vi "PSUSettingsMenu.vi"(8 "error in (no error)":errorcluster, 9 "PSU Calc":T1={"Low speed (km/s)"=2000.0, "High speed (km/s)"=3000.0, "Window (Delta-T)"=0.0, "Lower Cutoff"=0.0, "Multiplier"=0, "Low Charge (fC)"=2000.0, "High Charge (fC)"=2000.0, "High Mass (kg)"=2000.0, "Low Mass (kg)"=2000.0, "High Radius (µm) "=0.0, "Low Radius (µm)"=2000.0, "Exp. Voltage (MV)"=2000.0} {"Exp. Voltage (MV)" step=0.01 format="%#.6f"; "Window (Delta-T)" step=1.0 format="%#.0f"; "High Radius (µm)" min=0.0 max=1000.0; "High Mass (kg)" min=0.0 max=1.0; "High Charge (fC)" min=0.0 max=1000000000000.0; "High speed (km/s)" min=0.0 max=299790.0; "Low speed (km/s)" min=0.0 max=299790.0; "Low Charge (fC)" min=0.0 max=1000000000000.0; "Low Mass (kg)" min=0.0 max=1.0; "Low Radius (µm)" min=0.0 max=299792000.0; "Lower Cutoff" step=1.0 format="%#.0f"; "Multiplier" items=["1k", "10k"]}, 10 "sub vi?":bool, 11 "Enable":bool=TRUE) -> (0 "error out":errorcluster, 1 "OK":bool, 3 "Cancel 2":bool caption="Cancel")   [LabVIEW 2013]
doc: "Displays a standard dialog box that prompts users to enter information, such as a user name and password.\n--------------------\n\nThis Express VI is configured as follows:\n\nMessage to Display to the User:Please Enter Experiment Settings Information For Database Storage.\nThe inputs are: \nNumber: Please Enter Group ID\nText Entry Box: Please Enter Tags:\nText Entry Box: Please Enter Experiment Description:"
uses:
  Controls/PSU Calc.ctl
  <vilib>/Utility/miscctls.llb/LVPointTypeDef.ctl
  Global Variables/PSU updated.vi
  Sub-Polymorphic/post_psu.vi
  <vilib>/addons/database/_DB Variant To Data/Database Variant To Data.xnode
panel:
  in  "Accept All Particles":bool caption="OK2"
  out "Dust Density\n(g/cc)":dbl
  in  "Variable 2":enum32{"Velocity", "Charge", "Mass"}(radio)
  in  "Variable 1":enum32{"Velocity", "Charge", "Mass"}(radio)
  in  "PSU update":bool caption="OK2"
  in  "Cancel":bool
  in  "OK1":bool
  # "Please Enter PSU Settings For Storage in the CCLDAS Database."
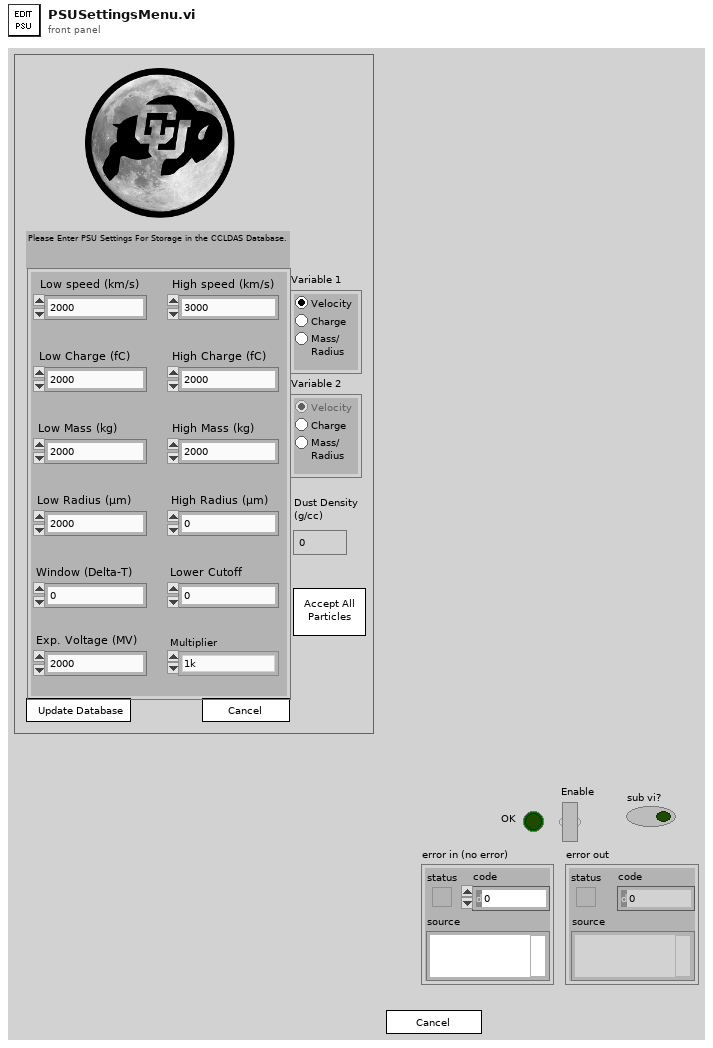
[diagram p1: front panel]
types:
  T1 = typedef "PSU Calc.ctl" = cluster{"Low speed (km/s)":dbl, "High speed (km/s)":dbl, "Window (Delta-T)":dbl, "Lower Cutoff":dbl, "Multiplier":u16, "Low Charge (fC)":dbl, "High Charge (fC)":dbl, "High Mass (kg)":dbl, "Low Mass (kg)":dbl, "High Radius (µm) ":dbl, "Low Radius (µm)":dbl, "Exp. Voltage (MV)":dbl}
  T2 = typedef "LVPointTypeDef.ctl" = cluster{"Horizontal":i16, "Vertical":i16}
  T3 = enum32{"Invalid", "Standard", "Closed", "Hidden", "Minimized", "Maximized"}
  T4 = enum8{"Enabled", "Disabled", "Disabled and Grayed Out"}
  T5 = cluster{"Integer Timestamp":i64, "Max Velocity":dbl, "Min Velocity":dbl, "Max Charge":dbl, "Min Charge":dbl, "Max Mass":dbl, "Min Mass":dbl, "Variable 1":enum8{"Velocity", "Charge", "Mass"}, "Variable 2":enum8{"Velocity", "Charge", "Mass"}}
  T6 = cluster{"Integer Timestamp":dbl, "Max Velocity":dbl, "Min Velocity":dbl, "Max Charge":dbl, "Min Charge":dbl, "Max Mass":dbl, "Min Mass":dbl, "Variable 1":enum32{"Velocity", "Charge", "Mass", "Radius"}, "Variable 2":enum32{"Velocity", "Charge", "Mass", "Radius"}}
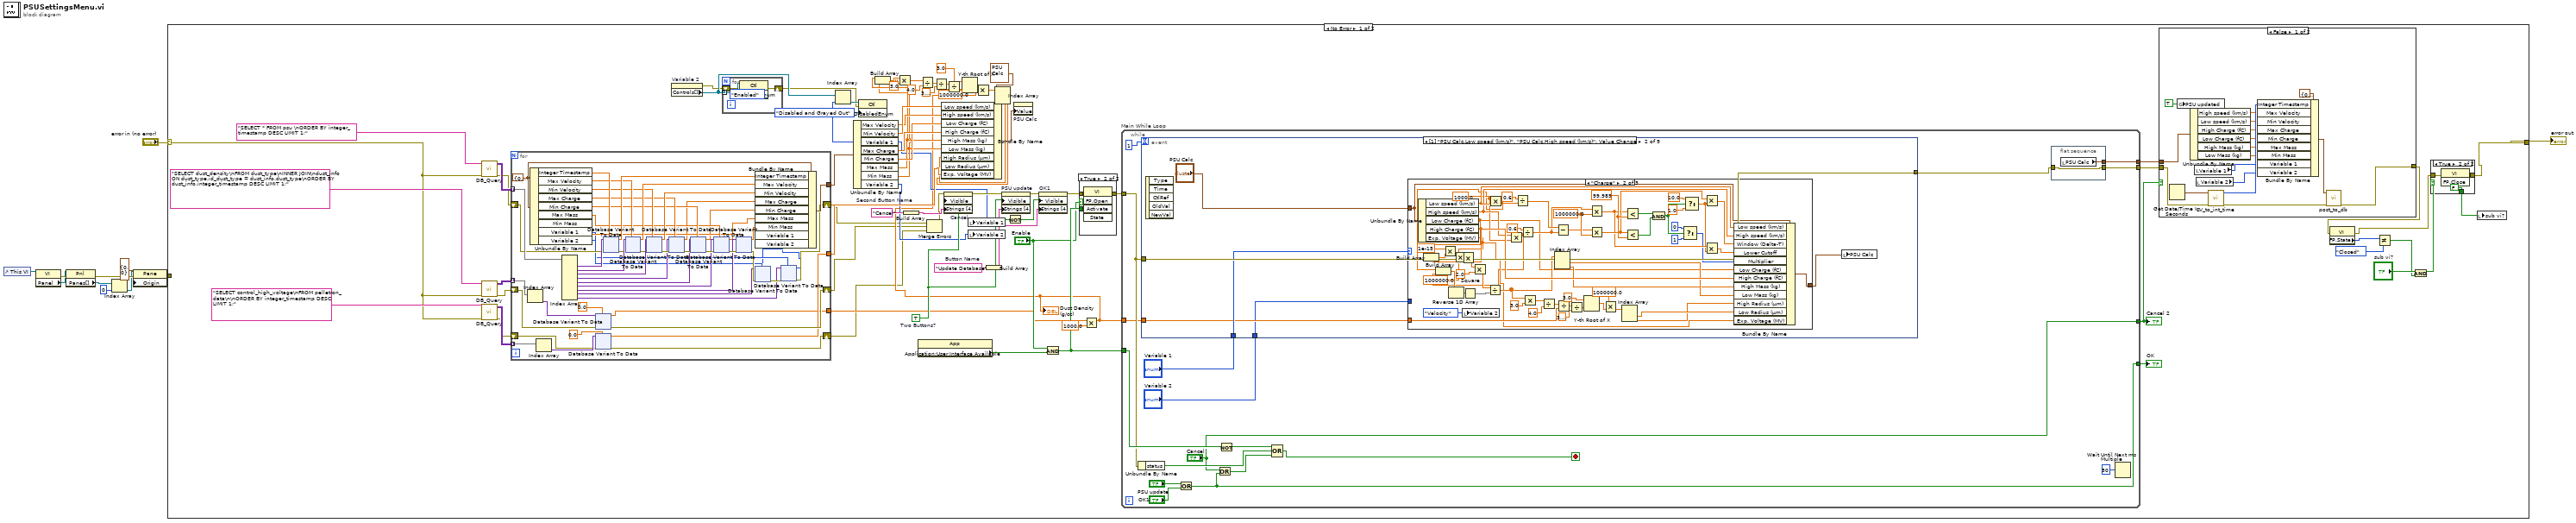
[diagram p0: block diagram]
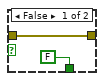
[diagram p2: hidden frame]
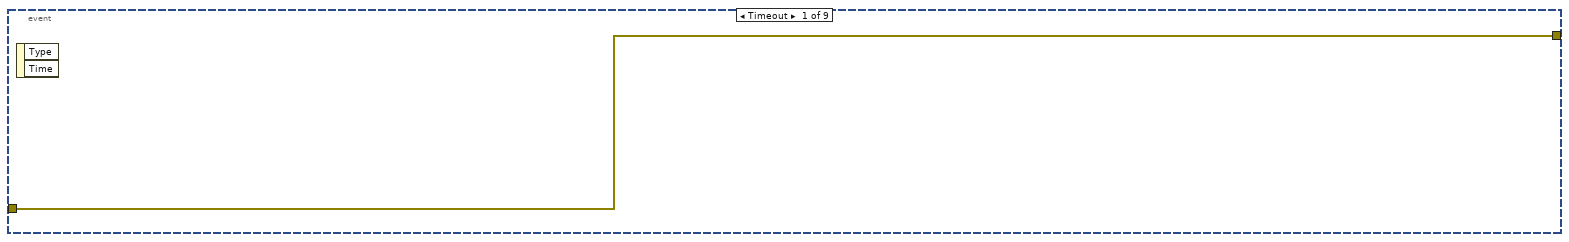
[diagram p5: hidden frame]
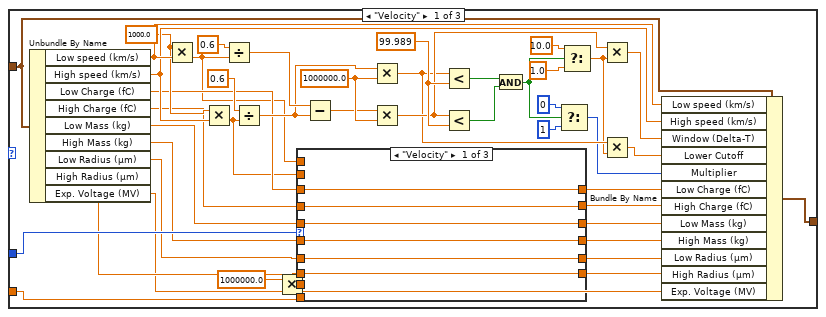
[diagram p6: hidden frame]
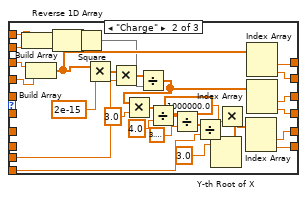
[diagram p7: hidden frame]
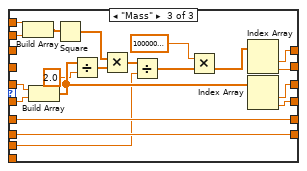
[diagram p8: hidden frame]
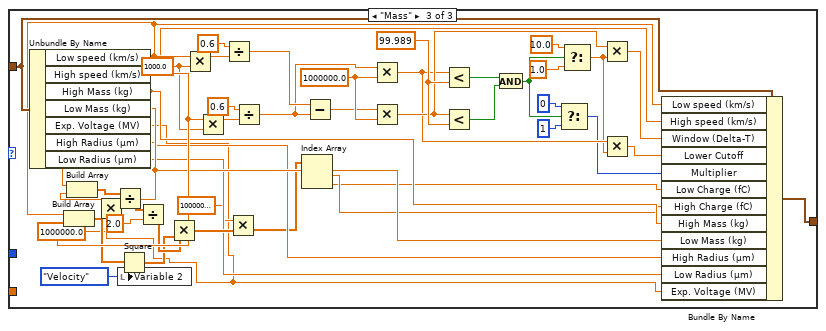
[diagram p9: hidden frame]
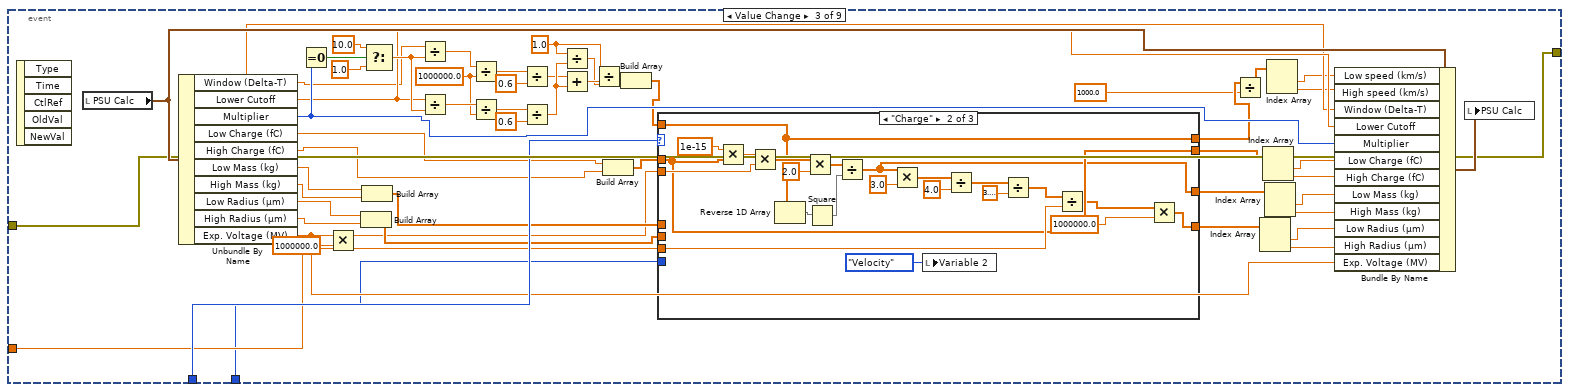
[diagram p10: hidden frame]
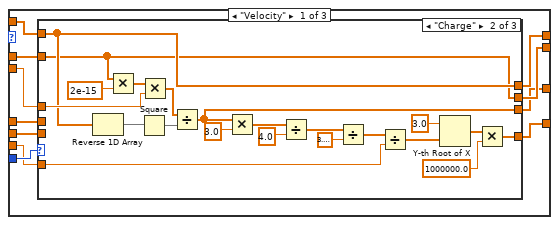
[diagram p11: hidden frame]
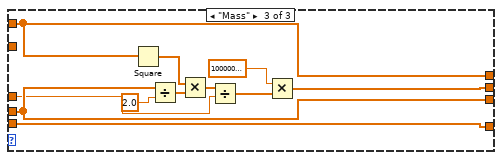
[diagram p13: hidden frame]
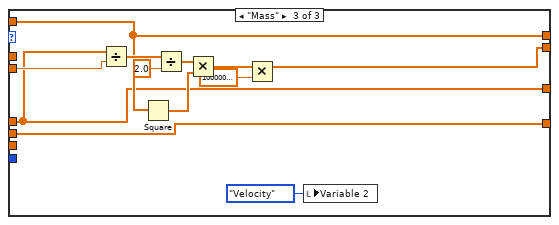
[diagram p14: hidden frame]
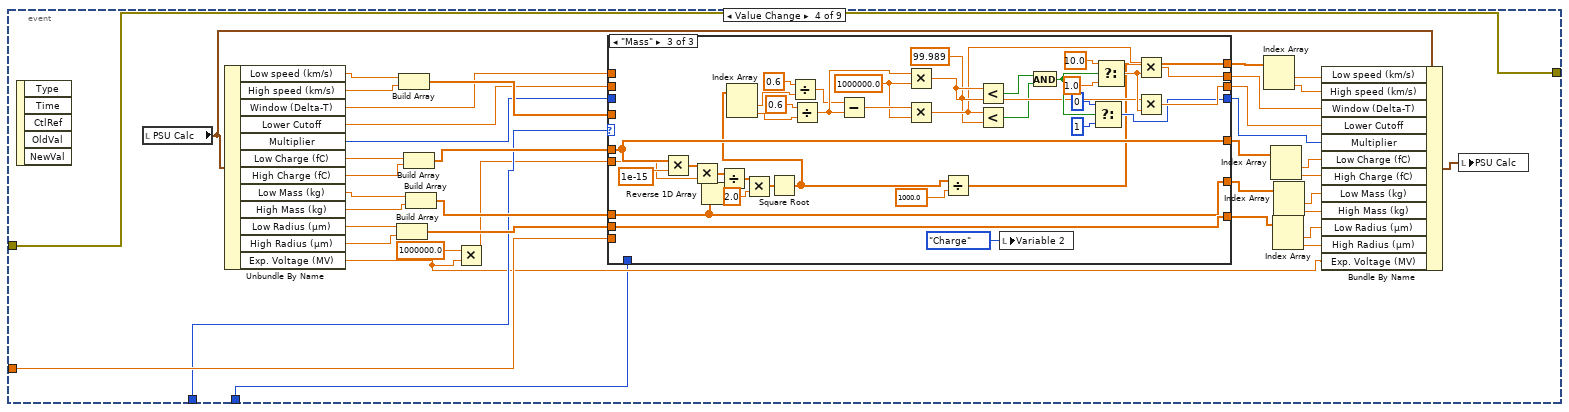
[diagram p15: hidden frame]
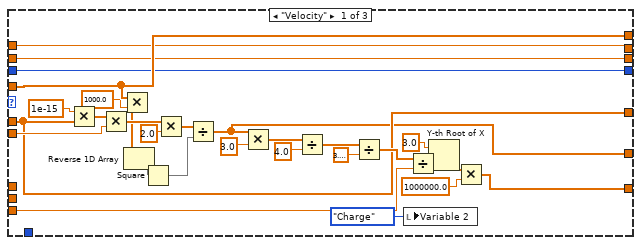
[diagram p16: hidden frame]
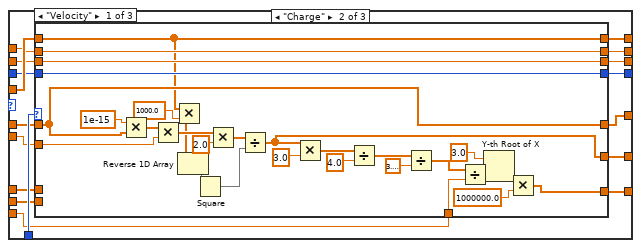
[diagram p17: hidden frame]
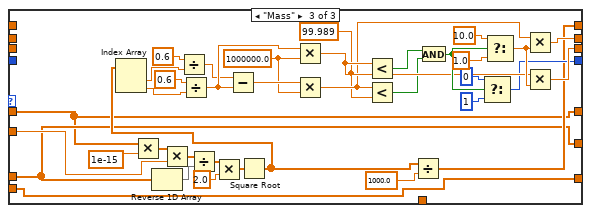
[diagram p19: hidden frame]
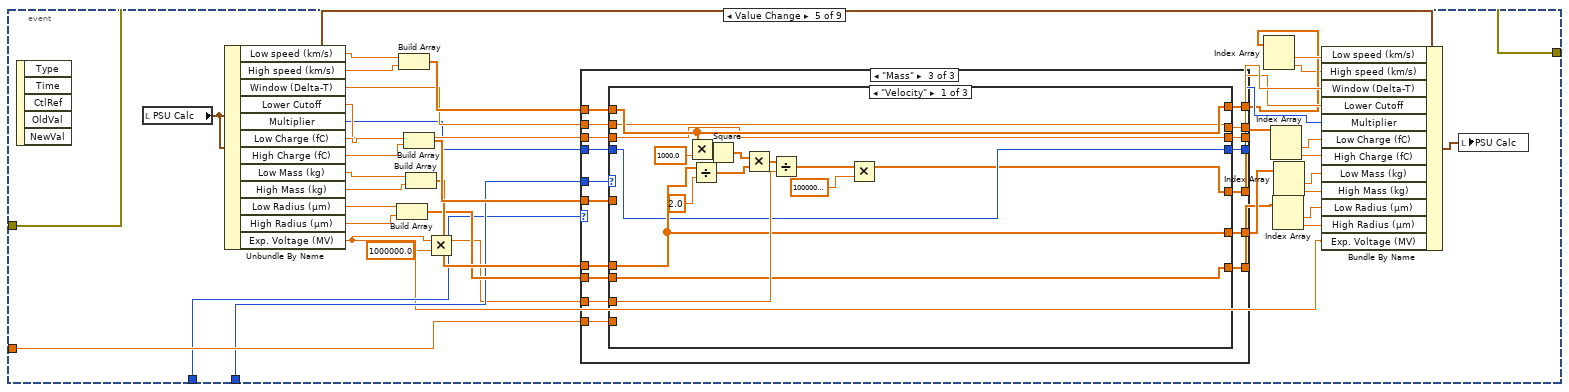
[diagram p20: hidden frame]
diagram:
  n1 = control-ref of="This VI"() -> (w9:refnum<vi>)
  n2 = property class="VI"(reference=w9) -> (error out=w8:errorcluster, "Panel"=w7:refnum<vi>)  [unwired: 1 in, 1 out]
  n3 = property class="Pnl"(reference=w7, error in=w8) -> (error out=w6:errorcluster, "Panes[]"=w5:refnum<vi>[])  [unwired: 1 out]
  n4 = Index Array(array=w5, index=0) -> (element=w3:refnum<vi>)
  n5 = property class="Pane"(reference=w3, error in=w6, "Origin"=T2 {"Horizontal"=0, "Vertical"=0}) -> (error out=w1:errorcluster)  [unwired: 1 out]
  n6 = case shown="No Error" "error in (no error)" {
    selector: "error in (no error)" -> [w13 w1720]
    tunnel: [w36 w1720] -> w10
    tunnel: w1 -> [_ _]
    frame No Error {
      w80 = "Cancel"  # Second Button Name
      w82 = "Update Database"  # Button Name
      w74 = TRUE  # Two Buttons?
      n7 = call "DB_Query.vi"("error in (no error)"=w13, "Parameterized Query"="SELECT * FROM psu \nORDER BY integer_timestamp DESC LIMIT 1;" ("SQL query")) -> ("error out"=w17:errorcluster, "Results"=w19:variant[][])  [unwired: 7 in, 1 out]
      n8 = call "DB_Query.vi"("error in (no error)"=w13, "Parameterized Query"="SELECT dust_density\nFROM dust_type\nINNER JOIN\ndust_info ON dust_type.id_dust_type = dust_info.dust_type\nORDER BY dust_info.integer_timestamp DESC LIMIT 1;" ("SQL query")) -> ("error out"=w18:errorcluster, "Results"=w21:variant[][])  [unwired: 7 in, 1 out]
      n9 = call "DB_Query.vi"("error in (no error)"=w13, "Parameterized Query"="SELECT control_high_voltage\nFROM pelletron_data\n\nORDER BY integer_timestamp DESC LIMIT 1;" ("SQL query")) -> ("error out"=w12:errorcluster, "Results"=w23:variant[][])  [unwired: 7 in, 1 out]
      n10 = for {
        tunnel: w19 -> [w168] mode=indexing
        shift-right: [w127] -> w14
        shift-left: w17 -> [w164]
        tunnel: [w163] -> w73
        tunnel: w21 -> [w137] mode=indexing
        shift-right: [w131] -> w15
        shift-left: w18 -> [w132]
        tunnel: w23 -> [w136] mode=indexing
        shift-right: [w130] -> w16
        shift-left: w12 -> [w133]
        tunnel: [w119] -> w60
        tunnel: [w117] -> w26
        w158 = T6 {"Integer Timestamp"=0.0, "Max Velocity"=0.0, "Min Velocity"=0.0, "Max Charge"=0.0, "Min Charge"=0.0, "Max Mass"=0.0, "Min Mass"=0.0, "Variable 1"=enum."Velocity", "Variable 2"=enum."Velocity"} ("PSU settings")
        n11 = Index Array(array=w137) -> (element=w135:variant)  [unwired: 1 in]
        n12 = Unbundle By Name(w158) -> ("Integer Timestamp"=w162:dbl, "Max Velocity"=w159:dbl, "Min Velocity"=w156:dbl, "Max Charge"=w145:dbl, "Min Charge"=w144:dbl, "Max Mass"=w143:dbl, "Min Mass"=w142:dbl, "Variable 1"=w124:enum32{"Velocity", "Charge", "Mass", "Radius"}, "Variable 2"=w123:enum32{"Velocity", "Charge", "Mass", "Radius"})
        n13 = Index Array(array=w136) -> (element=w134:variant)  [unwired: 1 in]
        n14 = Index Array(array=w168) -> (element #1=w167:variant, element #2=w166:variant, element #3=w157:variant, element #4=w150:variant, element #5=w149:variant, element #6=w148:variant, element #7=w146:variant, element #8=w126:variant, element #9=w125:variant)  [unwired: 9 in]
        n15 = xnode "Database Variant To Data"("database variant"=w135, "error in (no error)"=w132, "type"=0.0) -> ("data"=w117:dbl, "error out"=w131:errorcluster)
        n16 = xnode "Database Variant To Data"("database variant"=w134, "error in (no error)"=w133, "type"=0.0) -> ("data"=w119:dbl, "error out"=w130:errorcluster)
        n17 = xnode "Database Variant To Data"("database variant"=w167, "error in"=w164, "type"=w162) -> ("data"=w161:dbl, "error out"=w165:errorcluster)
        n18 = xnode "Database Variant To Data"("database variant"=w166, "error in"=w165, "type"=w159) -> ("data"=w160:dbl, "error out"=w154:errorcluster)
        n19 = xnode "Database Variant To Data"("database variant"=w157, "error in"=w154, "type"=w156) -> ("data"=w155:dbl, "error out"=w151:errorcluster)
        n20 = xnode "Database Variant To Data"("database variant"=w150, "error in (no error)"=w151, "type"=w145) -> ("data"=w141:dbl, "error out"=w153:errorcluster)
        n21 = xnode "Database Variant To Data"("database variant"=w149, "error in (no error)"=w153, "type"=w144) -> ("data"=w140:dbl, "error out"=w152:errorcluster)
        n22 = xnode "Database Variant To Data"("database variant"=w148, "error in (no error)"=w152, "type"=w143) -> ("data"=w139:dbl, "error out"=w147:errorcluster)
        n23 = xnode "Database Variant To Data"("database variant"=w146, "error in (no error)"=w147, "type"=w142) -> ("data"=w138:dbl, "error out"=w128:errorcluster)
        n24 = xnode "Database Variant To Data"("database variant"=w126, "error in (no error)"=w128, "type"=w124) -> ("data"=w122:enum32{"Velocity", "Charge", "Mass", "Radius"}, "error out"=w129:errorcluster)
        n25 = xnode "Database Variant To Data"("database variant"=w125, "error in (no error)"=w129, "type"=w123) -> ("data"=w121:enum32{"Velocity", "Charge", "Mass", "Radius"}, "error out"=w127:errorcluster)
        n26 = Bundle By Name(cluster=w158, "Integer Timestamp"=w161, "Max Velocity"=w160, "Min Velocity"=w155, "Max Charge"=w141, "Min Charge"=w140, "Max Mass"=w139, "Min Mass"=w138, "Variable 1"=w122, "Variable 2"=w121) -> (w163:T6)
      }
      n27 = property on="Variable 2" class="RadioBtnsControl (strict)"() -> (error out=w42:errorcluster, "Controls[]"=w43:refnum<vi>[])  [unwired: 2 in, 1 out]
      n28 = for {
        tunnel: w43 -> [w98] mode=indexing
        shift-right: [w95] -> w41
        shift-left: w42 -> [w97]
        n29 = property class="Ctl"(reference=w98, error in=w97, "DisabledEnum"=T4."Enabled" ("Disabled")) -> (error out=w95:errorcluster)  [unwired: 1 out]
      }
      n30 = Unbundle By Name(w73) -> ("Max Velocity"=w69:dbl, "Min Velocity"=w70:dbl, "Variable 1"=w40:enum32{"Velocity", "Charge", "Mass", "Radius"}, "Max Charge"=w62:dbl, "Min Charge"=w61:dbl, "Max Mass"=w59:dbl, "Min Mass"=w58:dbl, "Variable 2"=w39:enum32{"Velocity", "Charge", "Mass", "Radius"})
      n31 = Index Array(array=w43, index=w40) -> (element=w64:refnum<vi>)
      n32 = property class="Ctl"(reference=w64, error in=w41, "DisabledEnum"=T4."Disabled and Grayed Out" ("Disabled")) -> ()  [unwired: 2 out]
      n33 = Build Array(w59, w58) -> (w57:dbl[])
      n34 = Multiply(x=w57, y=3.0 ("Min Mass")) -> (x*y=w55:dbl[])
      n35 = Build Array(w80) -> (w79:string[])
      n36 = property class="App"() -> ("Application:User Interface Available"=w84:bool)  [unwired: 2 in, 2 out]
      n37 = Divide(x=w55, y=4.0 ("Min Mass")) -> (x/y=w53:dbl[])
      n38 = Merge Errors(w14, w15, w16) -> (w65:errorcluster)
      n39 = Divide(x=w53, y=3.141592653589793) -> (x/y=w51:dbl[])
      n40 = property on="Cancel" class="Bool"(error in=w65, "Visible"=w74, "Strings [4]"=w79) -> (error out=w77:errorcluster)  [unwired: 1 in, 1 out]
      n41 = local write "Variable 1"(w40) -> ()
      n42 = local write "Variable 2"(w39) -> ()
      n43 = Build Array(w82) -> (w81:string[])
      n44 = property on="PSU update" class="Bool"(error in=w77, "Visible"=w74, "Strings [4]"=w81) -> (error out=w78:errorcluster)  [unwired: 1 in, 1 out]
      n45 = Not(x=w74) -> (.not. x?=w76:bool)
      n46 = property on="OK1" class="Bool"(error in=w78, "Visible"=w76, "Strings [4]"=w81) -> (error out=w83:errorcluster)  [unwired: 1 in, 1 out]
      n47 = And(x="Enable", y=w84) -> (x .and. y?=w38:bool)
      n48 = case shown="True" "Enable" {
        tunnel: [w91 w94] -> w85
        tunnel: w83 -> [w91 w93]
        tunnel: w38 -> [_ w92]
        frame False {
        }
        frame True {
          n49 = invoke class="VI" method="FP.Open"(error in=w93, "Activate"=w92) -> (error out=w94:errorcluster)  [unwired: 3 in, 4 out]
        }
      }
      n50 = Multiply(x=w26, y=1000.0) -> (x*y=w25:dbl)
      "Dust Density\n(g/cc)" <- w25
      n51 = Divide(x=w51, y=w25) -> (x/y=w50:dbl[])
      n52 = Y-th Root of X(1:w50, 2:3.0 ("Min Mass")) -> (0:w46:dbl[])
      n53 = Multiply(x=w46, y=1000000.0 ("Min Mass")) -> (x*y=w45:dbl[])
      n54 = Index Array(array=w45) -> (element #1=w49:dbl, element #2=w48:dbl)  [unwired: 2 in]
      n55 = Bundle By Name(cluster=T1 {"Low speed (km/s)"=2000.0, "High speed (km/s)"=3000.0, "Window (Delta-T)"=0.0, "Lower Cutoff"=0.0, "Multiplier"=0, "Low Charge (fC)"=0.0, "High Charge (fC)"=0.0, "High Mass (kg)"=0.0, "Low Mass (kg)"=0.0, "High Radius (µm) "=0.0, "Low Radius (µm)"=0.0, "Exp. Voltage (MV)"=0.0} ("PSU Calc"), "Low speed (km/s)"=w70, "High speed (km/s)"=w69, "Low Charge (fC)"=w61, "High Charge (fC)"=w62, "High Mass (kg)"=w59, "Low Mass (kg)"=w58, "High Radius (µm)"=w49, "Low Radius (µm)"=w48, "Exp. Voltage (MV)"=w60) -> (w72:T1)
      n56 = property on="PSU Calc" class="Clust (strict)"("Value"=w72) -> ()  [unwired: 2 in, 2 out]
      n57 = while "Main While Loop" {
        tunnel: [w536] -> w75
        tunnel: w38 -> [w534]
        tunnel: w85 -> [w528]
        tunnel: [w526] -> w67
        tunnel: ["Cancel"] -> w68
        tunnel: [w524] -> w66
        tunnel: w25 -> [w522]
        stop <- w530 stop-if-true
        n58 = Unbundle By Name(w528) -> ("status"=w531:bool)
        n59 = event shown="[1] \"PSU Calc.Low speed (km/s)\", \"PSU Calc.High speed (km/s)\": Value Change" {
          selector: _ -> [_ _ _ _ _ _ _ _ _]
          dyn-events: _ -> [_ _ _ _ _ _ _ _ _]
          timeout: 1 -> [_ _ _ _ _ _ _ _ _]
          tunnel: w528 -> [w541 w546 w804 w892 w1084 w1356 w1367 w1535 w1719]
          tunnel: [w541 w546 w804 w892 w1084 w1348 w1367 w1535 w1697] -> w525
          tunnel: "Variable 1" -> [_ w544 w785 w893 w1085 _ w1381 w1551 _]
          tunnel: w522 -> [_ w543 w778 w912 w1105 _ w1373 w1544 _]
          tunnel: "Variable 2" -> [_ w542 w754 w888 w1086 w1352 w1363 w1531 _]
          event Timeout {
            n60 = event-data() -> ()  [unwired: 1 in, 2 out]
          }
          event Value Change {
            n61 = event-data() -> ()  [unwired: 1 in, 5 out]
            n62 = case shown="\"Charge\"" w544 {
              tunnel: [w591 w707 w753] -> w547
              tunnel: "PSU Calc" -> [w590 w706 w752]
              tunnel: w543 -> [w550 w668 _]
              tunnel: w542 -> [w566 _ _]
              frame "Velocity" {
                w567 = 1000.0 ("x")
                w581 = 99.989
                w583 = 1000000.0 ("y")
                n63 = Unbundle By Name(w590) -> ("Low speed (km/s)"=w572:dbl, "High speed (km/s)"=w568:dbl, "Low Charge (fC)"=w565:dbl, "High Charge (fC)"=w563:dbl, "Low Mass (kg)"=w561:dbl, "High Mass (kg)"=w560:dbl, "Low Radius (µm)"=w557:dbl, "High Radius (µm)"=w555:dbl, "Exp. Voltage (MV)"=w553:dbl)
                n64 = Multiply(x=w567, y=w572) -> (x*y=w551:dbl)
                n65 = Multiply(x=w567, y=w568) -> (x*y=w552:dbl)
                n66 = Divide(x=0.6, y=w551) -> (x/y=w585:dbl)
                n67 = Divide(x=0.6, y=w552) -> (x/y=w584:dbl)
                n68 = Multiply(x=1000000.0, y=w553) -> (x*y=w549:dbl)
                n69 = case shown="\"Velocity\"" w566 {
                  tunnel: w565 -> [w597 w625 _]
                  tunnel: [w597 w624 w642] -> w564
                  tunnel: w563 -> [w596 w626 _]
                  tunnel: [w596 w619 w639] -> w562
                  tunnel: w561 -> [w595 _ w646]
                  tunnel: [w595 w623 w641] -> w559
                  tunnel: w560 -> [w594 _ w645]
                  tunnel: [w594 w622 w640] -> w558
                  tunnel: w557 -> [w593 _ w644]
                  tunnel: [w593 w621 w644] -> w556
                  tunnel: w555 -> [w592 _ w643]
                  tunnel: [w592 w620 w643] -> w554
                  tunnel: w549 -> [_ w615 w632]
                  tunnel: w552 -> [_ w627 w647]
                  tunnel: w551 -> [_ w628 w648]
                  tunnel: w550 -> [_ w602 _]
                  frame "Velocity" {
                  }
                  frame "Charge" {
                    n70 = Build Array(w628, w627) -> (w613:dbl[])
                    n71 = Build Array(w625, w626) -> (w618:dbl[])
                    n72 = Reverse 1D Array(array=w613) -> (reversed array=w598:dbl[])
                    n73 = Square(x=w598) -> (x^2=w612:dbl[])
                    n74 = Multiply(x=w618, y=2e-15 ("x")) -> (x*y=w616:dbl[])
                    n75 = Multiply(x=w616, y=w615) -> (x*y=w614:dbl[])
                    n76 = Divide(x=w614, y=w612) -> (x/y=w611:dbl[])
                    n77 = Multiply(x=w611, y=3.0 ("x")) -> (x*y=w609:dbl[])
                    n78 = Divide(x=w609, y=4.0 ("x")) -> (x/y=w608:dbl[])
                    n79 = Divide(x=w608, y=3.141592653589793) -> (x/y=w607:dbl[])
                    n80 = Divide(x=w607, y=w602) -> (x/y=w606:dbl[])
                    n81 = Y-th Root of X(1:w606, 2:3.0 ("x")) -> (0:w601:dbl[])
                    n82 = Multiply(x=w601, y=1000000.0 ("x")) -> (x*y=w600:dbl[])
                    n83 = Index Array(array=w600) -> (element #1=w621:dbl, element #2=w620:dbl)  [unwired: 2 in]
                    n84 = Index Array(array=w618) -> (element #1=w624:dbl, element #2=w619:dbl)  [unwired: 2 in]
                    n85 = Index Array(array=w611) -> (element #1=w623:dbl, element #2=w622:dbl)  [unwired: 2 in]
                  }
                  frame "Mass" {
                    n86 = Build Array(w648, w647) -> (w638:dbl[])
                    n87 = Build Array(w646, w645) -> (w637:dbl[])
                    n88 = Square(x=w638) -> (x^2=w634:dbl[])
                    n89 = Divide(x=w637, y=2.0 ("x")) -> (x/y=w635:dbl[])
                    n90 = Multiply(x=w634, y=w635) -> (x*y=w633:dbl[])
                    n91 = Divide(x=w633, y=w632) -> (x/y=w631:dbl[])
                    n92 = Multiply(x=1000000000000000.0, y=w631) -> (x*y=w630:dbl[])
                    n93 = Index Array(array=w630) -> (element #1=w642:dbl, element #2=w639:dbl)  [unwired: 2 in]
                    n94 = Index Array(array=w637) -> (element #1=w641:dbl, element #2=w640:dbl)  [unwired: 2 in]
                  }
                }
                n95 = Subtract(x=w585, y=w584) -> (x-y=w582:dbl)
                n96 = Multiply(x=w584, y=w583) -> (x*y=w575:dbl)
                n97 = Multiply(x=w582, y=w583) -> (x*y=w576:dbl)
                n98 = Less?(x=w575, y=w581) -> (x < y?=w580:bool)
                n99 = Less?(x=w576, y=w581) -> (x < y?=w579:bool)
                n100 = And(x=w580, y=w579) -> (x .and. y?=w573:bool)
                n101 = Select(t=u16 0 ("Multiplier"), s=w573, f=u16 1 ("Multiplier")) -> (s? t:f=w569:u16)
                n102 = Select(t=10.0, s=w573, f=1.0) -> (s? t:f=w574:dbl)
                n103 = Multiply(x=w576, y=w574) -> (x*y=w588:dbl)
                n104 = Multiply(x=w575, y=w574) -> (x*y=w589:dbl)
                n105 = Bundle By Name(cluster=w590, "Low speed (km/s)"=w572, "High speed (km/s)"=w568, "Window (Delta-T)"=w588, "Lower Cutoff"=w589, "Multiplier"=w569, "Low Charge (fC)"=w564, "High Charge (fC)"=w562, "Low Mass (kg)"=w559, "High Mass (kg)"=w558, "Low Radius (µm)"=w556, "High Radius (µm)"=w554, "Exp. Voltage (MV)"=w553) -> (w591:T1)
              }
              frame "Charge" {
                w656 = 1000.0 ("x")
                w697 = 99.989
                w699 = 1000000.0 ("y")
                n106 = Unbundle By Name(w706) -> ("Low speed (km/s)"=w680:dbl, "High speed (km/s)"=w679:dbl, "Low Charge (fC)"=w655:dbl, "High Charge (fC)"=w684:dbl, "Exp. Voltage (MV)"=w654:dbl)
                n107 = Build Array(w655, w684) -> (w683:dbl[])
                n108 = Multiply(x=1e-15, y=w683) -> (x*y=w660:dbl[])
                n109 = Multiply(x=w654, y=1000000.0) -> (x*y=w653:dbl)
                n110 = Multiply(x=w660, y=w653) -> (x*y=w682:dbl[])
                n111 = local write "Variable 2"(enum32{"Velocity", "Charge", "Mass"}."Velocity" ("Variable 2")) -> ()
                n112 = Multiply(x=w682, y=2.0) -> (x*y=w677:dbl[])
                n113 = Multiply(x=w656, y=w680) -> (x*y=w651:dbl)
                n114 = Multiply(x=w679, y=w656) -> (x*y=w650:dbl)
                n115 = Build Array(w651, w650) -> (w678:dbl[])
                n116 = Reverse 1D Array(array=w678) -> (reversed array=w649:dbl[])
                n117 = Square(x=w649) -> (x^2=w676:dbl[])
                n118 = Divide(x=w677, y=w676) -> (x/y=w673:dbl[])
                n119 = Divide(x=0.6, y=w651) -> (x/y=w701:dbl)
                n120 = Divide(x=0.6, y=w650) -> (x/y=w700:dbl)
                n121 = Multiply(x=w673, y=3.0) -> (x*y=w671:dbl[])
                n122 = Divide(x=w671, y=4.0) -> (x/y=w669:dbl[])
                n123 = Index Array(array=w673) -> (element #1=w675:dbl, element #2=w674:dbl)  [unwired: 2 in]
                n124 = Subtract(x=w701, y=w700) -> (x-y=w698:dbl)
                n125 = Divide(x=w669, y=w668) -> (x/y=w667:dbl[])
                n126 = Divide(x=w667, y=3.141592653589793) -> (x/y=w665:dbl[])
                n127 = Y-th Root of X(1:w665, 2:3.0) -> (0:w663:dbl[])
                n128 = Multiply(x=w700, y=w699) -> (x*y=w691:dbl)
                n129 = Multiply(x=w698, y=w699) -> (x*y=w692:dbl)
                n130 = Multiply(x=1000000.0, y=w663) -> (x*y=w658:dbl[])
                n131 = Index Array(array=w658) -> (element #1=w662:dbl, element #2=w661:dbl)  [unwired: 2 in]
                n132 = Less?(x=w691, y=w697) -> (x < y?=w696:bool)
                n133 = Less?(x=w692, y=w697) -> (x < y?=w695:bool)
                n134 = And(x=w696, y=w695) -> (x .and. y?=w689:bool)
                n135 = Select(t=u16 0 ("Multiplier"), s=w689, f=u16 1 ("Multiplier")) -> (s? t:f=w686:u16)
                n136 = Select(t=10.0, s=w689, f=1.0) -> (s? t:f=w690:dbl)
                n137 = Multiply(x=w692, y=w690) -> (x*y=w704:dbl)
                n138 = Multiply(x=w691, y=w690) -> (x*y=w705:dbl)
                n139 = Bundle By Name(cluster=w706, "Low speed (km/s)"=w680, "High speed (km/s)"=w679, "Window (Delta-T)"=w704, "Lower Cutoff"=w705, "Multiplier"=w686, "Low Charge (fC)"=w655, "High Charge (fC)"=w684, "High Mass (kg)"=w674, "Low Mass (kg)"=w675, "High Radius (µm)"=w661, "Low Radius (µm)"=w662, "Exp. Voltage (MV)"=w654) -> (w707:T1)
              }
              frame "Mass" {
                w711 = 1000.0 ("y")
                w743 = 99.989
                w745 = 1000000.0 ("y")
                n140 = Unbundle By Name(w752) -> ("Low speed (km/s)"=w728:dbl, "High speed (km/s)"=w727:dbl, "High Mass (kg)"=w722:dbl, "Low Mass (kg)"=w721:dbl, "Exp. Voltage (MV)"=w710:dbl, "High Radius (µm)"=w717:dbl, "Low Radius (µm)"=w716:dbl)
                n141 = Build Array(w728, w727) -> (w726:dbl[])
                n142 = Build Array(w722, w721) -> (w718:dbl[])
                n143 = Multiply(x=w710, y=1000000.0) -> (x*y=w709:dbl)
                n144 = Divide(x=w718, y=w709) -> (x/y=w730:dbl[])
                n145 = local write "Variable 2"(enum32{"Velocity", "Charge", "Mass"}."Velocity" ("Variable 2")) -> ()
                n146 = Square(x=w726) -> (x^2=w724:dbl[])
                n147 = Divide(x=w730, y=2.0) -> (x/y=w725:dbl[])
                n148 = Multiply(x=w725, y=w724) -> (x*y=w723:dbl[])
                n149 = Multiply(x=w728, y=w711) -> (x*y=w713:dbl)
                n150 = Multiply(x=w727, y=w711) -> (x*y=w712:dbl)
                n151 = Divide(x=0.6, y=w713) -> (x/y=w747:dbl)
                n152 = Multiply(x=1000000000000000.0, y=w723) -> (x*y=w715:dbl[])
                n153 = Divide(x=0.6, y=w712) -> (x/y=w746:dbl)
                n154 = Index Array(array=w715) -> (element #1=w720:dbl, element #2=w719:dbl)  [unwired: 2 in]
                n155 = Subtract(x=w747, y=w746) -> (x-y=w744:dbl)
                n156 = Multiply(x=w746, y=w745) -> (x*y=w737:dbl)
                n157 = Multiply(x=w744, y=w745) -> (x*y=w738:dbl)
                n158 = Less?(x=w737, y=w743) -> (x < y?=w742:bool)
                n159 = Less?(x=w738, y=w743) -> (x < y?=w741:bool)
                n160 = And(x=w742, y=w741) -> (x .and. y?=w735:bool)
                n161 = Select(t=u16 0 ("Multiplier"), s=w735, f=u16 1 ("Multiplier")) -> (s? t:f=w732:u16)
                n162 = Select(t=10.0, s=w735, f=1.0) -> (s? t:f=w736:dbl)
                n163 = Multiply(x=w738, y=w736) -> (x*y=w750:dbl)
                n164 = Multiply(x=w737, y=w736) -> (x*y=w751:dbl)
                n165 = Bundle By Name(cluster=w752, "Low speed (km/s)"=w728, "High speed (km/s)"=w727, "Window (Delta-T)"=w750, "Lower Cutoff"=w751, "Multiplier"=w732, "Low Charge (fC)"=w719, "High Charge (fC)"=w720, "High Mass (kg)"=w722, "Low Mass (kg)"=w721, "High Radius (µm)"=w717, "Low Radius (µm)"=w716, "Exp. Voltage (MV)"=w710) -> (w753:T1)
              }
            }
            n166 = local write "PSU Calc"(w547) -> ()
          }
          event Value Change {
            w797 = 1.0 ("x")
            w800 = 1000000.0 ("y")
            n167 = event-data() -> ()  [unwired: 1 in, 5 out]
            n168 = local read "PSU Calc"() -> (w806:T1)
            n169 = Unbundle By Name(w806) -> ("Window (Delta-T)"=w788:dbl, "Lower Cutoff"=w789:dbl, "Multiplier"=w791:u16, "Low Charge (fC)"=w781:dbl, "High Charge (fC)"=w780:dbl, "Low Mass (kg)"=w777:dbl, "High Mass (kg)"=w776:dbl, "Low Radius (µm)"=w775:dbl, "High Radius (µm)"=w774:dbl, "Exp. Voltage (MV)"=w757:dbl)
            n170 = Equal To 0?(x=w791) -> (x = 0?=w792:bool)
            n171 = Multiply(x=w757, y=1000000.0) -> (x*y=w756:dbl)
            n172 = Build Array(w775, w774) -> (w772:dbl[])
            n173 = Build Array(w777, w776) -> (w773:dbl[])
            n174 = Select(t=10.0, s=w792, f=1.0) -> (s? t:f=w790:dbl)
            n175 = Divide(x=w788, y=w790) -> (x/y=w803:dbl)
            n176 = Divide(x=w789, y=w790) -> (x/y=w801:dbl)
            n177 = Divide(x=w803, y=w800) -> (x/y=w795:dbl)
            n178 = Divide(x=w801, y=w800) -> (x/y=w798:dbl)
            n179 = Divide(x=w795, y=0.6) -> (x/y=w794:dbl)
            n180 = Divide(x=w798, y=0.6) -> (x/y=w796:dbl)
            n181 = Divide(x=w797, y=w796) -> (x/y=w783:dbl)
            n182 = Add(x=w794, y=w796) -> (x+y=w793:dbl)
            n183 = Divide(x=w797, y=w793) -> (x/y=w784:dbl)
            n184 = Build Array(w781, w780) -> (w779:dbl[])
            n185 = Build Array(w784, w783) -> (w782:dbl[])
            n186 = case shown="\"Charge\"" w785 {
              tunnel: w782 -> [w816 w863 w882]
              tunnel: w756 -> [w808 w869 w887]
              tunnel: w779 -> [w814 w862 _]
              tunnel: w778 -> [w807 w868 _]
              tunnel: w773 -> [w812 _ w880]
              tunnel: w772 -> [w810 _ w881]
              tunnel: [w815 w863 w882] -> w759
              tunnel: [w813 w862 w878] -> w769
              tunnel: [w811 w856 w880] -> w768
              tunnel: [w809 w858 w881] -> w767
              tunnel: w754 -> [w817 _ _]
              frame "Velocity" {
                n187 = case shown="\"Charge\"" w817 {
                  tunnel: w816 -> [w821 w825 w846]
                  tunnel: [w821 w825 w846] -> w815
                  tunnel: w814 -> [w820 w824 _]
                  tunnel: [w820 w824 w845] -> w813
                  tunnel: w812 -> [w819 _ w844]
                  tunnel: [w819 w826 w844] -> w811
                  tunnel: w810 -> [w818 _ w847]
                  tunnel: [w818 w823 w847] -> w809
                  tunnel: w808 -> [_ w828 w843]
                  tunnel: w807 -> [_ w827 _]
                  frame "Velocity" {
                  }
                  frame "Charge" {
                    n188 = Reverse 1D Array(array=w825) -> (reversed array=w822:dbl[])
                    n189 = Multiply(x=w824, y=2e-15 ("x")) -> (x*y=w830:dbl[])
                    n190 = Square(x=w822) -> (x^2=w832:dbl[])
                    n191 = Multiply(x=w830, y=w828) -> (x*y=w831:dbl[])
                    n192 = Divide(x=w831, y=w832) -> (x/y=w826:dbl[])
                    n193 = Multiply(x=w826, y=3.0 ("x")) -> (x*y=w834:dbl[])
                    n194 = Divide(x=w834, y=4.0 ("x")) -> (x/y=w835:dbl[])
                    n195 = Divide(x=w835, y=3.141592653589793) -> (x/y=w836:dbl[])
                    n196 = Divide(x=w836, y=w827) -> (x/y=w837:dbl[])
                    n197 = Y-th Root of X(1:w837, 2:3.0 ("x")) -> (0:w841:dbl[])
                    n198 = Multiply(x=w841, y=1000000.0 ("x")) -> (x*y=w823:dbl[])
                  }
                  frame "Mass" {
                    n199 = Square(x=w846) -> (x^2=w851:dbl[])
                    n200 = Divide(x=w844, y=2.0 ("x")) -> (x/y=w852:dbl[])
                    n201 = Multiply(x=w851, y=w852) -> (x*y=w850:dbl[])
                    n202 = Divide(x=w850, y=w843) -> (x/y=w849:dbl[])
                    n203 = Multiply(x=1000000000000000.0, y=w849) -> (x*y=w845:dbl[])
                  }
                }
              }
              frame "Charge" {
                n204 = Multiply(x=1e-15 ("Exp. Voltage (V)"), y=w862) -> (x*y=w860:dbl[])
                n205 = Multiply(x=w860, y=w869) -> (x*y=w867:dbl[])
                n206 = Reverse 1D Array(array=w863) -> (reversed array=w854:dbl[])
                n207 = Multiply(x=w867, y=2.0 ("Exp. Voltage (V)")) -> (x*y=w865:dbl[])
                n208 = Square(x=w854) -> (x^2=w864:dbl[])
                n209 = Divide(x=w865, y=w864) -> (x/y=w856:dbl[])
                n210 = Multiply(x=w856, y=3.0 ("Exp. Voltage (V)")) -> (x*y=w874:dbl[])
                n211 = local write "Variable 2"(enum32{"Velocity", "Charge", "Mass"}."Velocity" ("Variable 2")) -> ()
                n212 = Divide(x=w874, y=4.0 ("Exp. Voltage (V)")) -> (x/y=w872:dbl[])
                n213 = Divide(x=w872, y=3.141592653589793) -> (x/y=w870:dbl[])
                n214 = Divide(x=w870, y=w868) -> (x/y=w861:dbl[])
                n215 = Multiply(x=w861, y=1000000.0 ("Exp. Voltage (V)")) -> (x*y=w858:dbl[])
              }
              frame "Mass" {
                n216 = Divide(x=w880, y=w887) -> (x/y=w886:dbl[])
                n217 = Square(x=w882) -> (x^2=w883:dbl[])
                n218 = Divide(x=w886, y=2.0 ("Exp. Voltage (V)")) -> (x/y=w884:dbl[])
                n219 = Multiply(x=w884, y=w883) -> (x*y=w879:dbl[])
                n220 = Multiply(x=w879, y=1000000000000000.0 ("Exp. Voltage (V)")) -> (x*y=w878:dbl[])
                n221 = local write "Variable 2"(enum32{"Velocity", "Charge", "Mass"}."Velocity" ("Variable 2")) -> ()
              }
            }
            n222 = Divide(x=w759, y=1000.0 ("Exp. Voltage (V)")) -> (x/y=w760:dbl[])
            n223 = Index Array(array=w767) -> (element #1=w762:dbl, element #2=w761:dbl)  [unwired: 2 in]
            n224 = Index Array(array=w769) -> (element #1=w766:dbl, element #2=w765:dbl)  [unwired: 2 in]
            n225 = Index Array(array=w768) -> (element #1=w764:dbl, element #2=w763:dbl)  [unwired: 2 in]
            n226 = Index Array(array=w760) -> (element #1=w771:dbl, element #2=w770:dbl)  [unwired: 2 in]
            n227 = Bundle By Name(cluster=w806, "Low speed (km/s)"=w771, "High speed (km/s)"=w770, "Window (Delta-T)"=w788, "Lower Cutoff"=w789, "Multiplier"=w791, "Low Charge (fC)"=w766, "High Charge (fC)"=w765, "Low Mass (kg)"=w764, "High Mass (kg)"=w763, "Low Radius (µm)"=w762, "High Radius (µm)"=w761, "Exp. Voltage (MV)"=w757) -> (w805:T1)
            n228 = local write "PSU Calc"(w805) -> ()
          }
          event Value Change {
            n229 = event-data() -> ()  [unwired: 1 in, 5 out]
            n230 = local read "PSU Calc"() -> (w925:T1)
            n231 = Unbundle By Name(w925) -> ("Low speed (km/s)"=w924:dbl, "High speed (km/s)"=w923:dbl, "Window (Delta-T)"=w911:dbl, "Lower Cutoff"=w910:dbl, "Multiplier"=w909:u16, "Low Charge (fC)"=w921:dbl, "High Charge (fC)"=w920:dbl, "Low Mass (kg)"=w919:dbl, "High Mass (kg)"=w918:dbl, "Low Radius (µm)"=w917:dbl, "High Radius (µm)"=w916:dbl, "Exp. Voltage (MV)"=w891:dbl)
            n232 = Build Array(w917, w916) -> (w913:dbl[])
            n233 = Build Array(w924, w923) -> (w922:dbl[])
            n234 = Build Array(w921, w920) -> (w915:dbl[])
            n235 = Build Array(w919, w918) -> (w914:dbl[])
            n236 = Multiply(x=1000000.0, y=w891) -> (x*y=w890:dbl)
            n237 = case shown="\"Mass\"" w893 {
              tunnel: w922 -> [w936 w971 _]
              tunnel: w890 -> [w949 w957 w1054]
              tunnel: w915 -> [w943 w963 w1057]
              tunnel: w912 -> [w948 w956 _]
              tunnel: w914 -> [_ w961 w1052]
              tunnel: w913 -> [_ w959 w1080]
              tunnel: [w936 w970 w1047] -> w904
              tunnel: [w943 w962 w1057] -> w903
              tunnel: [w937 w960 w1052] -> w902
              tunnel: [w939 w958 w1080] -> w901
              tunnel: w911 -> [w935 w969 _]
              tunnel: w910 -> [w934 w967 _]
              tunnel: w909 -> [w933 w965 _]
              tunnel: [w935 w968 w1060] -> w908
              tunnel: [w934 w966 w1059] -> w907
              tunnel: [w933 w964 w1058] -> w906
              tunnel: w888 -> [_ w972 _]
              frame "Velocity" {
                n238 = Multiply(x=1e-15 ("Exp. Voltage (V)"), y=w943) -> (x*y=w941:dbl[])
                n239 = Multiply(x=w941, y=w949) -> (x*y=w947:dbl[])
                n240 = Multiply(x=w936, y=1000.0 ("Exp. Voltage (V)")) -> (x*y=w931:dbl[])
                n241 = Reverse 1D Array(array=w931) -> (reversed array=w927:dbl[])
                n242 = Square(x=w927) -> (x^2=w944:dbl[])
                n243 = Multiply(x=w947, y=2.0 ("Exp. Voltage (V)")) -> (x*y=w945:dbl[])
                n244 = Divide(x=w945, y=w944) -> (x/y=w937:dbl[])
                n245 = Multiply(x=w937, y=3.0 ("Exp. Voltage (V)")) -> (x*y=w954:dbl[])
                n246 = Divide(x=w954, y=4.0 ("Exp. Voltage (V)")) -> (x/y=w952:dbl[])
                n247 = Divide(x=w952, y=3.141592653589793) -> (x/y=w950:dbl[])
                n248 = local write "Variable 2"(enum32{"Velocity", "Charge", "Mass"}."Charge" ("Variable 2")) -> ()
                n249 = Divide(x=w950, y=w948) -> (x/y=w942:dbl[])
                n250 = Y-th Root of X(1:w942, 2:3.0 ("Exp. Voltage (V)")) -> (0:w929:dbl[])
                n251 = Multiply(x=w929, y=1000000.0 ("Exp. Voltage (V)")) -> (x*y=w939:dbl[])
              }
              frame "Charge" {
                n252 = case shown="\"Velocity\"" w972 {
                  tunnel: w971 -> [w976 w1007 _]
                  tunnel: [w976 w1007 w1011] -> w970
                  tunnel: w969 -> [w1000 w1006 _]
                  tunnel: [w1000 w1006 w1024] -> w968
                  tunnel: w967 -> [w999 w1005 _]
                  tunnel: [w999 w1005 w1023] -> w966
                  tunnel: w965 -> [w998 w1004 _]
                  tunnel: [w998 w1004 w1022] -> w964
                  tunnel: w963 -> [w981 w1003 w1009]
                  tunnel: [w981 w1003 w1009] -> w962
                  tunnel: w961 -> [_ w1002 w1010]
                  tunnel: [w977 w1002 w1010] -> w960
                  tunnel: w959 -> [_ w1001 w1012]
                  tunnel: [w978 w1001 w1012] -> w958
                  tunnel: w957 -> [w980 _ w1014]
                  tunnel: w956 -> [w979 _ _]
                  frame "Velocity" {
                    n253 = Multiply(x=1e-15 ("Exp. Voltage (V)"), y=w981) -> (x*y=w986:dbl[])
                    n254 = Multiply(x=w986, y=w980) -> (x*y=w991:dbl[])
                    n255 = Multiply(x=w976, y=1000.0 ("Exp. Voltage (V)")) -> (x*y=w983:dbl[])
                    n256 = Reverse 1D Array(array=w983) -> (reversed array=w973:dbl[])
                    n257 = Square(x=w973) -> (x^2=w988:dbl[])
                    n258 = Multiply(x=w991, y=2.0 ("Exp. Voltage (V)")) -> (x*y=w989:dbl[])
                    n259 = Divide(x=w989, y=w988) -> (x/y=w977:dbl[])
                    n260 = Multiply(x=w977, y=3.0 ("Exp. Voltage (V)")) -> (x*y=w996:dbl[])
                    n261 = Divide(x=w996, y=4.0 ("Exp. Voltage (V)")) -> (x/y=w994:dbl[])
                    n262 = Divide(x=w994, y=3.141592653589793) -> (x/y=w992:dbl[])
                    n263 = Divide(x=w992, y=w979) -> (x/y=w987:dbl[])
                    n264 = Y-th Root of X(1:w987, 2:3.0 ("Exp. Voltage (V)")) -> (0:w975:dbl[])
                    n265 = Multiply(x=w975, y=1000000.0 ("Exp. Voltage (V)")) -> (x*y=w978:dbl[])
                  }
                  frame "Charge" {
                  }
                  frame "Mass" {
                    w1031 = 99.989
                    w1029 = 1000000.0 ("y")
                    n266 = Multiply(x=w1009, y=1e-15 ("x")) -> (x*y=w1020:dbl[])
                    n267 = Reverse 1D Array(array=w1010) -> (reversed array=w1008:dbl[])
                    n268 = Multiply(x=w1020, y=w1014) -> (x*y=w1019:dbl[])
                    n269 = Divide(x=w1019, y=w1008) -> (x/y=w1018:dbl[])
                    n270 = Multiply(x=w1018, y=2.0 ("x")) -> (x*y=w1016:dbl[])
                    n271 = Square Root(x=w1016) -> (sqrt(x)=w1013:dbl[])
                    n272 = Index Array(array=w1013) -> (element #1=w1042:dbl, element #2=w1043:dbl)  [unwired: 2 in]
                    n273 = Divide(x=0.6, y=w1042) -> (x/y=w1027:dbl)
                    n274 = Divide(x=0.6, y=w1043) -> (x/y=w1028:dbl)
                    n275 = Subtract(x=w1027, y=w1028) -> (x-y=w1030:dbl)
                    n276 = Multiply(x=w1028, y=w1029) -> (x*y=w1037:dbl)
                    n277 = Multiply(x=w1030, y=w1029) -> (x*y=w1036:dbl)
                    n278 = Less?(x=w1037, y=w1031) -> (x < y?=w1032:bool)
                    n279 = Less?(x=w1036, y=w1031) -> (x < y?=w1033:bool)
                    n280 = Divide(x=w1013, y=1000.0 ("x")) -> (x/y=w1011:dbl[])
                    n281 = And(x=w1032, y=w1033) -> (x .and. y?=w1039:bool)
                    n282 = Select(t=u16 0 ("Multiplier"), s=w1039, f=u16 1 ("Multiplier")) -> (s? t:f=w1022:u16)
                    n283 = Select(t=10.0, s=w1039, f=1.0) -> (s? t:f=w1038:dbl)
                    n284 = Multiply(x=w1036, y=w1038) -> (x*y=w1024:dbl)
                    n285 = Multiply(x=w1037, y=w1038) -> (x*y=w1023:dbl)
                  }
                }
              }
              frame "Mass" {
                w1067 = 99.989
                w1065 = 1000000.0 ("y")
                n286 = Multiply(x=w1057, y=1e-15 ("x")) -> (x*y=w1055:dbl[])
                n287 = Multiply(x=w1055, y=w1054) -> (x*y=w1053:dbl[])
                n288 = Reverse 1D Array(array=w1052) -> (reversed array=w1044:dbl[])
                n289 = Divide(x=w1053, y=w1044) -> (x/y=w1051:dbl[])
                n290 = Multiply(x=w1051, y=2.0 ("x")) -> (x*y=w1049:dbl[])
                n291 = Square Root(x=w1049) -> (sqrt(x)=w1046:dbl[])
                n292 = Index Array(array=w1046) -> (element #1=w1078:dbl, element #2=w1079:dbl)  [unwired: 2 in]
                n293 = Divide(x=0.6, y=w1078) -> (x/y=w1063:dbl)
                n294 = Divide(x=0.6, y=w1079) -> (x/y=w1064:dbl)
                n295 = Subtract(x=w1063, y=w1064) -> (x-y=w1066:dbl)
                n296 = Multiply(x=w1064, y=w1065) -> (x*y=w1073:dbl)
                n297 = Multiply(x=w1066, y=w1065) -> (x*y=w1072:dbl)
                n298 = Divide(x=w1046, y=1000.0 ("x")) -> (x/y=w1047:dbl[])
                n299 = Less?(x=w1073, y=w1067) -> (x < y?=w1068:bool)
                n300 = Less?(x=w1072, y=w1067) -> (x < y?=w1069:bool)
                n301 = local write "Variable 2"(enum32{"Velocity", "Charge", "Mass"}."Charge" ("Variable 2")) -> ()
                n302 = And(x=w1068, y=w1069) -> (x .and. y?=w1075:bool)
                n303 = Select(t=u16 0 ("Multiplier"), s=w1075, f=u16 1 ("Multiplier")) -> (s? t:f=w1058:u16)
                n304 = Select(t=10.0, s=w1075, f=1.0) -> (s? t:f=w1074:dbl)
                n305 = Multiply(x=w1072, y=w1074) -> (x*y=w1060:dbl)
                n306 = Multiply(x=w1073, y=w1074) -> (x*y=w1059:dbl)
              }
            }
            n307 = Index Array(array=w904) -> (element #1=w905:dbl, element #2=w898:dbl)  [unwired: 2 in]
            n308 = Index Array(array=w903) -> (element #1=w900:dbl, element #2=w899:dbl)  [unwired: 2 in]
            n309 = Index Array(array=w901) -> (element #1=w895:dbl, element #2=w894:dbl)  [unwired: 2 in]
            n310 = Index Array(array=w902) -> (element #1=w897:dbl, element #2=w896:dbl)  [unwired: 2 in]
            n311 = Bundle By Name(cluster=w925, "Low speed (km/s)"=w905, "High speed (km/s)"=w898, "Window (Delta-T)"=w908, "Lower Cutoff"=w907, "Multiplier"=w906, "Low Charge (fC)"=w900, "High Charge (fC)"=w899, "Low Mass (kg)"=w897, "High Mass (kg)"=w896, "Low Radius (µm)"=w895, "High Radius (µm)"=w894, "Exp. Voltage (MV)"=w891) -> (w926:T1)
            n312 = local write "PSU Calc"(w926) -> ()
          }
          event Value Change {
            n313 = event-data() -> ()  [unwired: 1 in, 5 out]
            n314 = local read "PSU Calc"() -> (w1118:T1)
            n315 = Unbundle By Name(w1118) -> ("Low speed (km/s)"=w1117:dbl, "High speed (km/s)"=w1116:dbl, "Window (Delta-T)"=w1104:dbl, "Lower Cutoff"=w1103:dbl, "Multiplier"=w1102:u16, "Low Charge (fC)"=w1114:dbl, "High Charge (fC)"=w1113:dbl, "Low Mass (kg)"=w1112:dbl, "High Mass (kg)"=w1111:dbl, "Low Radius (µm)"=w1110:dbl, "High Radius (µm)"=w1109:dbl, "Exp. Voltage (MV)"=w1083:dbl)
            n316 = Build Array(w1110, w1109) -> (w1106:dbl[])
            n317 = Build Array(w1117, w1116) -> (w1115:dbl[])
            n318 = Build Array(w1114, w1113) -> (w1108:dbl[])
            n319 = Build Array(w1112, w1111) -> (w1107:dbl[])
            n320 = Multiply(x=w1083, y=1000000.0) -> (x*y=w1082:dbl)
            n321 = case shown="\"Mass\"" w1085 {
              tunnel: w1115 -> [w1136 w1222 w1288]
              tunnel: w1108 -> [w1135 w1221 w1287]
              tunnel: w1107 -> [w1134 w1220 w1286]
              tunnel: w1106 -> [w1133 w1219 w1285]
              tunnel: w1082 -> [w1132 w1218 w1284]
              tunnel: w1105 -> [w1131 w1217 w1283]
              tunnel: w1104 -> [w1130 w1216 w1282]
              tunnel: w1103 -> [w1129 w1215 w1281]
              tunnel: w1102 -> [w1128 w1214 w1280]
              tunnel: [w1127 w1213 w1279] -> w1101
              tunnel: [w1126 w1212 w1278] -> w1100
              tunnel: [w1125 w1211 w1277] -> w1099
              tunnel: [w1124 w1210 w1276] -> w1097
              tunnel: [w1123 w1209 w1275] -> w1096
              tunnel: [w1122 w1208 w1274] -> w1095
              tunnel: [w1121 w1207 w1273] -> w1094
              tunnel: w1086 -> [w1120 w1206 w1272]
              frame "Charge" {
                n322 = case shown="\"Mass\"" w1120 {
                  tunnel: w1136 -> [w1143 w1169 _]
                  tunnel: w1132 -> [w1156 _ w1179]
                  tunnel: w1135 -> [w1150 w1168 w1182]
                  tunnel: w1131 -> [w1155 _ _]
                  tunnel: w1134 -> [_ w1167 w1177]
                  tunnel: w1133 -> [_ w1166 w1205]
                  tunnel: [w1143 w1169 w1173] -> w1124
                  tunnel: [w1150 w1168 w1182] -> w1123
                  tunnel: [w1144 w1167 w1177] -> w1122
                  tunnel: [w1146 w1166 w1205] -> w1121
                  tunnel: w1130 -> [w1142 w1165 _]
                  tunnel: w1129 -> [w1141 w1164 _]
                  tunnel: w1128 -> [w1140 w1163 _]
                  tunnel: [w1142 w1165 w1185] -> w1127
                  tunnel: [w1141 w1164 w1184] -> w1126
                  tunnel: [w1140 w1163 w1183] -> w1125
                  frame "Velocity" {
                    n323 = Multiply(x=1e-15 ("Exp. Voltage (V)"), y=w1150) -> (x*y=w1148:dbl[])
                    n324 = Multiply(x=w1148, y=w1156) -> (x*y=w1154:dbl[])
                    n325 = Multiply(x=w1143, y=1000.0 ("Exp. Voltage (V)")) -> (x*y=w1139:dbl[])
                    n326 = Reverse 1D Array(array=w1139) -> (reversed array=w1137:dbl[])
                    n327 = Square(x=w1137) -> (x^2=w1151:dbl[])
                    n328 = Multiply(x=w1154, y=2.0 ("Exp. Voltage (V)")) -> (x*y=w1152:dbl[])
                    n329 = Divide(x=w1152, y=w1151) -> (x/y=w1144:dbl[])
                    n330 = Multiply(x=w1144, y=3.0 ("Exp. Voltage (V)")) -> (x*y=w1161:dbl[])
                    n331 = Divide(x=w1161, y=4.0 ("Exp. Voltage (V)")) -> (x/y=w1159:dbl[])
                    n332 = Divide(x=w1159, y=3.141592653589793) -> (x/y=w1157:dbl[])
                    n333 = Divide(x=w1157, y=w1155) -> (x/y=w1149:dbl[])
                    n334 = Multiply(x=w1149, y=1000000.0 ("Exp. Voltage (V)")) -> (x*y=w1146:dbl[])
                  }
                  frame "Charge" {
                  }
                  frame "Mass" {
                    w1192 = 99.989
                    w1190 = 1000000.0 ("y")
                    n335 = Multiply(x=w1182, y=1e-15 ("x")) -> (x*y=w1180:dbl[])
                    n336 = Multiply(x=w1180, y=w1179) -> (x*y=w1178:dbl[])
                    n337 = Reverse 1D Array(array=w1177) -> (reversed array=w1170:dbl[])
                    n338 = Divide(x=w1178, y=w1170) -> (x/y=w1176:dbl[])
                    n339 = Multiply(x=w1176, y=2.0 ("x")) -> (x*y=w1174:dbl[])
                    n340 = Square Root(x=w1174) -> (sqrt(x)=w1172:dbl[])
                    n341 = Index Array(array=w1172) -> (element #1=w1203:dbl, element #2=w1204:dbl)  [unwired: 2 in]
                    n342 = Divide(x=0.6, y=w1203) -> (x/y=w1188:dbl)
                    n343 = Divide(x=0.6, y=w1204) -> (x/y=w1189:dbl)
                    n344 = Subtract(x=w1188, y=w1189) -> (x-y=w1191:dbl)
                    n345 = Multiply(x=w1189, y=w1190) -> (x*y=w1198:dbl)
                    n346 = Multiply(x=w1191, y=w1190) -> (x*y=w1197:dbl)
                    n347 = Divide(x=w1172, y=1000.0 ("x")) -> (x/y=w1173:dbl[])
                    n348 = Less?(x=w1198, y=w1192) -> (x < y?=w1193:bool)
                    n349 = Less?(x=w1197, y=w1192) -> (x < y?=w1194:bool)
                    n350 = And(x=w1193, y=w1194) -> (x .and. y?=w1200:bool)
                    n351 = Select(t=u16 0 ("Multiplier"), s=w1200, f=u16 1 ("Multiplier")) -> (s? t:f=w1183:u16)
                    n352 = Select(t=10.0, s=w1200, f=1.0) -> (s? t:f=w1199:dbl)
                    n353 = Multiply(x=w1197, y=w1199) -> (x*y=w1185:dbl)
                    n354 = Multiply(x=w1198, y=w1199) -> (x*y=w1184:dbl)
                  }
                }
              }
              frame "Velocity" {
                n355 = case shown="\"Charge\"" w1206 {
                  tunnel: w1222 -> [w1229 w1236 w1261]
                  tunnel: w1218 -> [_ w1249 w1259]
                  tunnel: w1221 -> [w1228 w1243 _]
                  tunnel: w1217 -> [_ w1248 _]
                  tunnel: w1220 -> [w1227 _ w1260]
                  tunnel: w1219 -> [w1226 _ w1268]
                  tunnel: [w1229 w1236 w1261] -> w1210
                  tunnel: [w1228 w1243 w1258] -> w1209
                  tunnel: [w1227 w1237 w1260] -> w1208
                  tunnel: [w1226 w1239 w1268] -> w1207
                  tunnel: w1216 -> [w1225 w1235 w1271]
                  tunnel: w1215 -> [w1224 w1234 w1270]
                  tunnel: w1214 -> [w1223 w1233 w1269]
                  tunnel: [w1225 w1235 w1271] -> w1213
                  tunnel: [w1224 w1234 w1270] -> w1212
                  tunnel: [w1223 w1233 w1269] -> w1211
                  frame "Velocity" {
                  }
                  frame "Charge" {
                    n356 = Multiply(x=1e-15 ("Exp. Voltage (V)"), y=w1243) -> (x*y=w1241:dbl[])
                    n357 = Multiply(x=w1241, y=w1249) -> (x*y=w1247:dbl[])
                    n358 = Multiply(x=w1236, y=1000.0 ("Exp. Voltage (V)")) -> (x*y=w1232:dbl[])
                    n359 = Reverse 1D Array(array=w1232) -> (reversed array=w1230:dbl[])
                    n360 = Square(x=w1230) -> (x^2=w1244:dbl[])
                    n361 = Multiply(x=w1247, y=2.0 ("Exp. Voltage (V)")) -> (x*y=w1245:dbl[])
                    n362 = Divide(x=w1245, y=w1244) -> (x/y=w1237:dbl[])
                    n363 = Multiply(x=w1237, y=3.0 ("Exp. Voltage (V)")) -> (x*y=w1254:dbl[])
                    n364 = Divide(x=w1254, y=4.0 ("Exp. Voltage (V)")) -> (x/y=w1252:dbl[])
                    n365 = Divide(x=w1252, y=3.141592653589793) -> (x/y=w1250:dbl[])
                    n366 = Divide(x=w1250, y=w1248) -> (x/y=w1242:dbl[])
                    n367 = Multiply(x=w1242, y=1000000.0 ("Exp. Voltage (V)")) -> (x*y=w1239:dbl[])
                  }
                  frame "Mass" {
                    n368 = Divide(x=w1260, y=w1259) -> (x/y=w1267:dbl[])
                    n369 = Multiply(x=w1261, y=1000.0 ("Exp. Voltage (V)")) -> (x*y=w1257:dbl[])
                    n370 = Square(x=w1257) -> (x^2=w1264:dbl[])
                    n371 = Divide(x=w1267, y=2.0 ("Exp. Voltage (V)")) -> (x/y=w1265:dbl[])
                    n372 = Multiply(x=w1265, y=w1264) -> (x*y=w1263:dbl[])
                    n373 = Multiply(x=w1263, y=1000000000000000.0 ("Exp. Voltage (V)")) -> (x*y=w1258:dbl[])
                  }
                }
              }
              frame "Mass" {
                n374 = case shown="\"Velocity\"" w1272 {
                  tunnel: w1288 -> [w1294 _ w1347]
                  tunnel: w1284 -> [w1298 w1311 _]
                  tunnel: w1287 -> [_ w1312 w1346]
                  tunnel: w1283 -> [_ _ _]
                  tunnel: w1286 -> [w1295 w1315 w1345]
                  tunnel: w1285 -> [w1296 w1314 w1344]
                  tunnel: [w1294 w1307 w1347] -> w1276
                  tunnel: [w1290 w1312 w1346] -> w1275
                  tunnel: [w1295 w1315 w1345] -> w1274
                  tunnel: [w1296 w1314 w1344] -> w1273
                  tunnel: w1282 -> [w1293 _ w1343]
                  tunnel: w1281 -> [w1292 _ w1342]
                  tunnel: w1280 -> [w1291 _ w1341]
                  tunnel: [w1293 w1308 w1343] -> w1279
                  tunnel: [w1292 w1309 w1342] -> w1278
                  tunnel: [w1291 w1310 w1341] -> w1277
                  frame "Velocity" {
                    n375 = Multiply(x=w1294, y=1000.0 ("Lower Cutoff")) -> (x*y=w1301:dbl[])
                    n376 = Divide(x=w1295, y=2.0 ("Lower Cutoff")) -> (x/y=w1302:dbl[])
                    n377 = Square(x=w1301) -> (x^2=w1303:dbl[])
                    n378 = Multiply(x=w1303, y=w1302) -> (x*y=w1299:dbl[])
                    n379 = Divide(x=w1299, y=w1298) -> (x/y=w1297:dbl[])
                    n380 = Multiply(x=w1297, y=1000000000000000.0 ("Lower Cutoff")) -> (x*y=w1290:dbl[])
                  }
                  frame "Charge" {
                    w1328 = 99.989
                    w1326 = 1000000.0 ("y")
                    n381 = Multiply(x=w1312, y=1e-15 ("x")) -> (x*y=w1320:dbl[])
                    n382 = Multiply(x=w1320, y=w1311) -> (x*y=w1319:dbl[])
                    n383 = Reverse 1D Array(array=w1315) -> (reversed array=w1305:dbl[])
                    n384 = Divide(x=w1319, y=w1305) -> (x/y=w1318:dbl[])
                    n385 = Multiply(x=w1318, y=2.0 ("x")) -> (x*y=w1316:dbl[])
                    n386 = Square Root(x=w1316) -> (sqrt(x)=w1313:dbl[])
                    n387 = Index Array(array=w1313) -> (element #1=w1339:dbl, element #2=w1340:dbl)  [unwired: 2 in]
                    n388 = Divide(x=0.6, y=w1339) -> (x/y=w1324:dbl)
                    n389 = Divide(x=0.6, y=w1340) -> (x/y=w1325:dbl)
                    n390 = Subtract(x=w1324, y=w1325) -> (x-y=w1327:dbl)
                    n391 = Multiply(x=w1325, y=w1326) -> (x*y=w1334:dbl)
                    n392 = Multiply(x=w1327, y=w1326) -> (x*y=w1333:dbl)
                    n393 = Less?(x=w1334, y=w1328) -> (x < y?=w1329:bool)
                    n394 = Less?(x=w1333, y=w1328) -> (x < y?=w1330:bool)
                    n395 = Divide(x=w1313, y=1000.0 ("x")) -> (x/y=w1307:dbl[])
                    n396 = And(x=w1329, y=w1330) -> (x .and. y?=w1336:bool)
                    n397 = Select(t=u16 0 ("Multiplier"), s=w1336, f=u16 1 ("Multiplier")) -> (s? t:f=w1310:u16)
                    n398 = Select(t=10.0, s=w1336, f=1.0) -> (s? t:f=w1335:dbl)
                    n399 = Multiply(x=w1333, y=w1335) -> (x*y=w1308:dbl)
                    n400 = Multiply(x=w1334, y=w1335) -> (x*y=w1309:dbl)
                  }
                  frame "Mass" {
                  }
                }
              }
            }
            n401 = Index Array(array=w1097) -> (element #1=w1098:dbl, element #2=w1091:dbl)  [unwired: 2 in]
            n402 = Index Array(array=w1096) -> (element #1=w1093:dbl, element #2=w1092:dbl)  [unwired: 2 in]
            n403 = Index Array(array=w1094) -> (element #1=w1088:dbl, element #2=w1087:dbl)  [unwired: 2 in]
            n404 = Index Array(array=w1095) -> (element #1=w1090:dbl, element #2=w1089:dbl)  [unwired: 2 in]
            n405 = Bundle By Name(cluster=w1118, "Low speed (km/s)"=w1098, "High speed (km/s)"=w1091, "Window (Delta-T)"=w1101, "Lower Cutoff"=w1100, "Multiplier"=w1099, "Low Charge (fC)"=w1093, "High Charge (fC)"=w1092, "Low Mass (kg)"=w1090, "High Mass (kg)"=w1089, "Low Radius (µm)"=w1088, "High Radius (µm)"=w1087, "Exp. Voltage (MV)"=w1083) -> (w1119:T1)
            n406 = local write "PSU Calc"(w1119) -> ()
          }
          event "Variable 1": Value Change {
            n407 = event-data() -> ("OldVal"=w1353:enum32{"Velocity", "Charge", "Mass"}, "NewVal"=w1355:enum32{"Velocity", "Charge", "Mass"})  [unwired: 1 in, 3 out]
            n408 = property on="Variable 2" class="RadioBtnsControl (strict)"(error in=w1356) -> (error out=w1357:errorcluster, "Controls[]"=w1362:refnum<vi>[])  [unwired: 1 in, 1 out]
            n409 = Index Array(array=w1362, index=w1353) -> (element=w1361:refnum<vi>)
            n410 = Index Array(array=w1362, index=w1355) -> (element=w1360:refnum<vi>)
            n411 = property class="Ctl"(reference=w1361, error in=w1357, "DisabledEnum"=T4."Enabled" ("Disabled")) -> (error out=w1350:errorcluster)  [unwired: 1 out]
            n412 = property class="Ctl"(reference=w1360, error in=w1357, "DisabledEnum"=T4."Disabled and Grayed Out" ("Disabled")) -> (error out=w1349:errorcluster)  [unwired: 1 out]
            n413 = Equal?(x=w1355, y=w1352) -> (x = y?=w1354:bool)
            n414 = Select(t=w1353, s=w1354, f=w1352) -> (s? t:f=w1351:enum32{"Velocity", "Charge", "Mass"})
            n415 = Merge Errors(w1350, w1349) -> (w1348:errorcluster)
            n416 = local write "Variable 2"(w1351) -> ()
          }
          event Value Change {
            n417 = event-data() -> ()  [unwired: 1 in, 5 out]
            n418 = local read "PSU Calc"() -> (w1407:T1)
            n419 = Unbundle By Name(w1407) -> ("Low speed (km/s)"=w1406:dbl, "High speed (km/s)"=w1405:dbl, "Window (Delta-T)"=w1398:dbl, "Lower Cutoff"=w1397:dbl, "Multiplier"=w1396:u16, "Low Charge (fC)"=w1403:dbl, "High Charge (fC)"=w1402:dbl, "Low Mass (kg)"=w1401:dbl, "High Mass (kg)"=w1400:dbl, "Exp. Voltage (MV)"=w1366:dbl)  [unwired: 2 out]
            n420 = Build Array(w1406, w1405) -> (w1404:dbl[])
            n421 = Build Array(w1403, w1402) -> (w1399:dbl[])
            n422 = Build Array(w1401, w1400) -> (w1380:dbl[])
            n423 = Multiply(x=1000000.0, y=w1366) -> (x*y=w1365:dbl)
            n424 = Multiply(x=w1380, y=3.0 ("x")) -> (x*y=w1378:dbl[])
            n425 = Divide(x=w1378, y=4.0 ("x")) -> (x/y=w1376:dbl[])
            n426 = case shown="\"Velocity\"" w1381 {
              tunnel: w1404 -> [w1418 _ w1473]
              tunnel: w1365 -> [w1412 w1435 w1461]
              tunnel: w1399 -> [_ w1438 w1465]
              tunnel: w1380 -> [w1420 w1433 w1462]
              tunnel: [w1418 w1428 w1472] -> w1391
              tunnel: [w1410 w1438 w1464] -> w1390
              tunnel: [w1420 w1433 w1463] -> w1389
              tunnel: w1398 -> [w1424 _ w1471]
              tunnel: w1397 -> [w1423 _ w1469]
              tunnel: w1396 -> [w1422 _ w1467]
              tunnel: [w1424 w1441 w1470] -> w1395
              tunnel: [w1423 w1440 w1468] -> w1394
              tunnel: [w1422 w1439 w1466] -> w1393
              tunnel: w1363 -> [_ _ w1474]
              frame "Velocity" {
                n427 = Multiply(x=w1418, y=1000.0 ("Lower Cutoff")) -> (x*y=w1415:dbl[])
                n428 = Divide(x=w1420, y=2.0 ("Lower Cutoff")) -> (x/y=w1416:dbl[])
                n429 = Square(x=w1415) -> (x^2=w1417:dbl[])
                n430 = Multiply(x=w1417, y=w1416) -> (x*y=w1413:dbl[])
                n431 = Divide(x=w1413, y=w1412) -> (x/y=w1411:dbl[])
                n432 = Multiply(x=1000000000000000.0 ("Lower Cutoff"), y=w1411) -> (x*y=w1410:dbl[])
                n433 = local write "Variable 2"(enum32{"Velocity", "Charge", "Mass"}."Mass" ("Variable 2")) -> ()
              }
              frame "Charge" {
                w1448 = 99.989
                w1446 = 1000000.0 ("y")
                n434 = Multiply(x=w1438, y=1e-15 ("x")) -> (x*y=w1436:dbl[])
                n435 = Multiply(x=w1436, y=w1435) -> (x*y=w1434:dbl[])
                n436 = Reverse 1D Array(array=w1433) -> (reversed array=w1425:dbl[])
                n437 = Divide(x=w1434, y=w1425) -> (x/y=w1432:dbl[])
                n438 = Multiply(x=w1432, y=2.0 ("x")) -> (x*y=w1430:dbl[])
                n439 = Square Root(x=w1430) -> (sqrt(x)=w1427:dbl[])
                n440 = Index Array(array=w1427) -> (element #1=w1459:dbl, element #2=w1460:dbl)  [unwired: 2 in]
                n441 = Divide(x=0.6, y=w1459) -> (x/y=w1444:dbl)
                n442 = Divide(x=0.6, y=w1460) -> (x/y=w1445:dbl)
                n443 = Subtract(x=w1444, y=w1445) -> (x-y=w1447:dbl)
                n444 = Multiply(x=w1445, y=w1446) -> (x*y=w1454:dbl)
                n445 = Multiply(x=w1447, y=w1446) -> (x*y=w1453:dbl)
                n446 = Divide(x=w1427, y=1000.0) -> (x/y=w1428:dbl[])
                n447 = Less?(x=w1454, y=w1448) -> (x < y?=w1449:bool)
                n448 = Less?(x=w1453, y=w1448) -> (x < y?=w1450:bool)
                n449 = local write "Variable 2"(enum32{"Velocity", "Charge", "Mass"}."Mass" ("Variable 2")) -> ()
                n450 = And(x=w1449, y=w1450) -> (x .and. y?=w1456:bool)
                n451 = Select(t=u16 0 ("Multiplier"), s=w1456, f=u16 1 ("Multiplier")) -> (s? t:f=w1439:u16)
                n452 = Select(t=10.0, s=w1456, f=1.0) -> (s? t:f=w1455:dbl)
                n453 = Multiply(x=w1453, y=w1455) -> (x*y=w1441:dbl)
                n454 = Multiply(x=w1454, y=w1455) -> (x*y=w1440:dbl)
              }
              frame "Mass" {
                n455 = case shown="\"Charge\"" w1474 {
                  tunnel: w1473 -> [w1477 _ w1530]
                  tunnel: [w1477 w1491 w1530] -> w1472
                  tunnel: w1471 -> [w1481 _ w1529]
                  tunnel: [w1481 w1505 w1529] -> w1470
                  tunnel: w1469 -> [w1480 _ w1528]
                  tunnel: [w1480 w1504 w1528] -> w1468
                  tunnel: w1467 -> [w1479 _ w1527]
                  tunnel: [w1479 w1503 w1527] -> w1466
                  tunnel: w1465 -> [_ w1494 w1526]
                  tunnel: [w1482 w1494 w1526] -> w1464
                  tunnel: [w1475 w1492 w1525] -> w1463
                  tunnel: w1462 -> [w1475 w1492 w1525]
                  tunnel: w1461 -> [w1483 w1493 _]
                  frame "Velocity" {
                    n456 = Multiply(x=w1477, y=1000.0 ("x")) -> (x*y=w1478:dbl[])
                    n457 = Square(x=w1478) -> (x^2=w1487:dbl[])
                    n458 = Divide(x=w1475, y=2.0 ("x")) -> (x/y=w1488:dbl[])
                    n459 = Multiply(x=w1487, y=w1488) -> (x*y=w1486:dbl[])
                    n460 = Divide(x=w1486, y=w1483) -> (x/y=w1485:dbl[])
                    n461 = Multiply(x=1000000000000000.0, y=w1485) -> (x*y=w1482:dbl[])
                  }
                  frame "Charge" {
                    w1518 = 99.989
                    w1520 = 1000000.0 ("y")
                    n462 = Multiply(x=w1494, y=1e-15 ("x")) -> (x*y=w1501:dbl[])
                    n463 = Multiply(x=w1501, y=w1493) -> (x*y=w1500:dbl[])
                    n464 = Reverse 1D Array(array=w1492) -> (reversed array=w1490:dbl[])
                    n465 = Divide(x=w1500, y=w1490) -> (x/y=w1499:dbl[])
                    n466 = Multiply(x=w1499, y=2.0 ("x")) -> (x*y=w1497:dbl[])
                    n467 = Square Root(x=w1497) -> (sqrt(x)=w1495:dbl[])
                    n468 = Index Array(array=w1495) -> (element #1=w1507:dbl, element #2=w1506:dbl)  [unwired: 2 in]
                    n469 = Divide(x=0.6, y=w1507) -> (x/y=w1522:dbl)
                    n470 = Divide(x=0.6, y=w1506) -> (x/y=w1521:dbl)
                    n471 = Subtract(x=w1522, y=w1521) -> (x-y=w1519:dbl)
                    n472 = Multiply(x=w1521, y=w1520) -> (x*y=w1512:dbl)
                    n473 = Multiply(x=w1519, y=w1520) -> (x*y=w1513:dbl)
                    n474 = Less?(x=w1512, y=w1518) -> (x < y?=w1517:bool)
                    n475 = Less?(x=w1513, y=w1518) -> (x < y?=w1516:bool)
                    n476 = Divide(x=w1495, y=1000.0 ("x")) -> (x/y=w1491:dbl[])
                    n477 = And(x=w1517, y=w1516) -> (x .and. y?=w1510:bool)
                    n478 = Select(t=u16 0 ("Multiplier"), s=w1510, f=u16 1 ("Multiplier")) -> (s? t:f=w1503:u16)
                    n479 = Select(t=10.0, s=w1510, f=1.0) -> (s? t:f=w1511:dbl)
                    n480 = Multiply(x=w1513, y=w1511) -> (x*y=w1505:dbl)
                    n481 = Multiply(x=w1512, y=w1511) -> (x*y=w1504:dbl)
                  }
                  frame "Mass" {
                  }
                }
              }
            }
            n482 = Divide(x=w1376, y=3.141592653589793) -> (x/y=w1374:dbl[])
            n483 = Divide(x=w1374, y=w1373) -> (x/y=w1372:dbl[])
            n484 = Y-th Root of X(1:w1372, 2:3.0 ("x")) -> (0:w1370:dbl[])
            n485 = Multiply(x=w1370, y=1000000.0 ("x")) -> (x*y=w1368:dbl[])
            n486 = Index Array(array=w1391) -> (element #1=w1392:dbl, element #2=w1386:dbl)  [unwired: 2 in]
            n487 = Index Array(array=w1390) -> (element #1=w1388:dbl, element #2=w1387:dbl)  [unwired: 2 in]
            n488 = Index Array(array=w1368) -> (element #1=w1383:dbl, element #2=w1382:dbl)  [unwired: 2 in]
            n489 = Index Array(array=w1389) -> (element #1=w1385:dbl, element #2=w1384:dbl)  [unwired: 2 in]
            n490 = Bundle By Name(cluster=w1407, "Low speed (km/s)"=w1392, "High speed (km/s)"=w1386, "Window (Delta-T)"=w1395, "Lower Cutoff"=w1394, "Multiplier"=w1393, "Low Charge (fC)"=w1388, "High Charge (fC)"=w1387, "Low Mass (kg)"=w1385, "High Mass (kg)"=w1384, "Low Radius (µm)"=w1383, "High Radius (µm)"=w1382, "Exp. Voltage (MV)"=w1366) -> (w1408:T1)
            n491 = local write "PSU Calc"(w1408) -> ()
          }
          event Value Change {
            n492 = event-data() -> ()  [unwired: 1 in, 5 out]
            n493 = local read "PSU Calc"() -> (w1575:T1)
            n494 = Unbundle By Name(w1575) -> ("Low speed (km/s)"=w1574:dbl, "High speed (km/s)"=w1573:dbl, "Window (Delta-T)"=w1568:dbl, "Lower Cutoff"=w1567:dbl, "Multiplier"=w1566:u16, "Low Charge (fC)"=w1571:dbl, "High Charge (fC)"=w1570:dbl, "Low Radius (µm)"=w1543:dbl, "High Radius (µm)"=w1542:dbl, "Exp. Voltage (MV)"=w1534:dbl)  [unwired: 2 out]
            n495 = Multiply(x=w1534, y=1000000.0) -> (x*y=w1533:dbl)
            n496 = Build Array(w1574, w1573) -> (w1572:dbl[])
            n497 = Build Array(w1571, w1570) -> (w1569:dbl[])
            n498 = Build Array(w1543, w1542) -> (w1539:dbl[])
            n499 = Divide(x=w1539, y=1000000.0 ("x")) -> (x/y=w1537:dbl[])
            n500 = Power Of X(1:w1537, 2:3.0 ("x")) -> (0:w1540:dbl[])
            n501 = Divide(x=w1540, y=3.0 ("x")) -> (x/y=w1549:dbl[])
            n502 = Multiply(x=w1549, y=4.0 ("x")) -> (x*y=w1547:dbl[])
            n503 = Multiply(x=w1547, y=3.141592653589793) -> (x*y=w1545:dbl[])
            n504 = Multiply(x=w1545, y=w1544) -> (x*y=w1541:dbl[])
            n505 = case shown="\"Velocity\"" w1551 {
              tunnel: w1572 -> [w1586 _ w1640]
              tunnel: w1533 -> [w1580 w1601 w1630]
              tunnel: w1569 -> [_ w1604 w1632]
              tunnel: w1541 -> [w1588 w1599 w1629]
              tunnel: [w1586 w1595 w1639] -> w1561
              tunnel: [w1578 w1604 w1631] -> w1560
              tunnel: [w1588 w1599 w1628] -> w1559
              tunnel: w1568 -> [w1592 _ w1638]
              tunnel: w1567 -> [w1591 _ w1636]
              tunnel: w1566 -> [w1590 _ w1634]
              tunnel: [w1592 w1607 w1637] -> w1565
              tunnel: [w1591 w1606 w1635] -> w1564
              tunnel: [w1590 w1605 w1633] -> w1563
              tunnel: w1531 -> [_ _ w1627]
              frame "Velocity" {
                n506 = Multiply(x=w1586, y=1000.0 ("Lower Cutoff")) -> (x*y=w1583:dbl[])
                n507 = Divide(x=w1588, y=2.0 ("Lower Cutoff")) -> (x/y=w1584:dbl[])
                n508 = Square(x=w1583) -> (x^2=w1585:dbl[])
                n509 = Multiply(x=w1585, y=w1584) -> (x*y=w1581:dbl[])
                n510 = Divide(x=w1581, y=w1580) -> (x/y=w1579:dbl[])
                n511 = Multiply(x=1000000000000000.0 ("Lower Cutoff"), y=w1579) -> (x*y=w1578:dbl[])
                n512 = local write "Variable 2"(enum32{"Velocity", "Charge", "Mass"}."Mass" ("Variable 2")) -> ()
              }
              frame "Charge" {
                w1614 = 99.989
                w1612 = 1000000.0 ("y")
                n513 = Multiply(x=w1604, y=1e-15 ("x")) -> (x*y=w1602:dbl[])
                n514 = Multiply(x=w1602, y=w1601) -> (x*y=w1600:dbl[])
                n515 = Reverse 1D Array(array=w1599) -> (reversed array=w1593:dbl[])
                n516 = Divide(x=w1600, y=w1593) -> (x/y=w1598:dbl[])
                n517 = Multiply(x=w1598, y=2.0 ("x")) -> (x*y=w1596:dbl[])
                n518 = Square Root(x=w1596) -> (sqrt(x)=w1595:dbl[])
                n519 = Index Array(array=w1595) -> (element #1=w1625:dbl, element #2=w1626:dbl)  [unwired: 2 in]
                n520 = Divide(x=0.6, y=w1625) -> (x/y=w1610:dbl)
                n521 = Divide(x=0.6, y=w1626) -> (x/y=w1611:dbl)
                n522 = Subtract(x=w1610, y=w1611) -> (x-y=w1613:dbl)
                n523 = Multiply(x=w1611, y=w1612) -> (x*y=w1620:dbl)
                n524 = Multiply(x=w1613, y=w1612) -> (x*y=w1619:dbl)
                n525 = Less?(x=w1620, y=w1614) -> (x < y?=w1615:bool)
                n526 = Less?(x=w1619, y=w1614) -> (x < y?=w1616:bool)
                n527 = local write "Variable 2"(enum32{"Velocity", "Charge", "Mass"}."Mass" ("Variable 2")) -> ()
                n528 = And(x=w1615, y=w1616) -> (x .and. y?=w1622:bool)
                n529 = Select(t=u16 0 ("Multiplier"), s=w1622, f=u16 1 ("Multiplier")) -> (s? t:f=w1605:u16)
                n530 = Select(t=10.0, s=w1622, f=1.0) -> (s? t:f=w1621:dbl)
                n531 = Multiply(x=w1619, y=w1621) -> (x*y=w1607:dbl)
                n532 = Multiply(x=w1620, y=w1621) -> (x*y=w1606:dbl)
              }
              frame "Mass" {
                n533 = case shown="\"Mass\"" w1627 {
                  tunnel: w1640 -> [w1643 _ w1696]
                  tunnel: [w1643 w1657 w1696] -> w1639
                  tunnel: w1638 -> [w1647 _ w1695]
                  tunnel: [w1647 w1671 w1695] -> w1637
                  tunnel: w1636 -> [w1646 _ w1694]
                  tunnel: [w1646 w1670 w1694] -> w1635
                  tunnel: w1634 -> [w1645 _ w1693]
                  tunnel: [w1645 w1669 w1693] -> w1633
                  tunnel: w1632 -> [_ w1660 w1692]
                  tunnel: [w1648 w1660 w1692] -> w1631
                  tunnel: [w1641 w1658 w1691] -> w1628
                  tunnel: w1629 -> [w1641 w1658 w1691]
                  tunnel: w1630 -> [w1649 w1659 _]
                  frame "Velocity" {
                    n534 = Multiply(x=w1643, y=1000.0 ("x")) -> (x*y=w1644:dbl[])
                    n535 = Square(x=w1644) -> (x^2=w1653:dbl[])
                    n536 = Divide(x=w1641, y=2.0 ("x")) -> (x/y=w1654:dbl[])
                    n537 = Multiply(x=w1653, y=w1654) -> (x*y=w1652:dbl[])
                    n538 = Divide(x=w1652, y=w1649) -> (x/y=w1651:dbl[])
                    n539 = Multiply(x=1000000000000000.0, y=w1651) -> (x*y=w1648:dbl[])
                  }
                  frame "Charge" {
                    w1684 = 99.989
                    w1686 = 1000000.0 ("y")
                    n540 = Multiply(x=w1660, y=1e-15 ("x")) -> (x*y=w1667:dbl[])
                    n541 = Multiply(x=w1667, y=w1659) -> (x*y=w1666:dbl[])
                    n542 = Reverse 1D Array(array=w1658) -> (reversed array=w1656:dbl[])
                    n543 = Divide(x=w1666, y=w1656) -> (x/y=w1665:dbl[])
                    n544 = Multiply(x=w1665, y=2.0 ("x")) -> (x*y=w1663:dbl[])
                    n545 = Square Root(x=w1663) -> (sqrt(x)=w1661:dbl[])
                    n546 = Index Array(array=w1661) -> (element #1=w1673:dbl, element #2=w1672:dbl)  [unwired: 2 in]
                    n547 = Divide(x=0.6, y=w1673) -> (x/y=w1688:dbl)
                    n548 = Divide(x=0.6, y=w1672) -> (x/y=w1687:dbl)
                    n549 = Subtract(x=w1688, y=w1687) -> (x-y=w1685:dbl)
                    n550 = Multiply(x=w1687, y=w1686) -> (x*y=w1678:dbl)
                    n551 = Multiply(x=w1685, y=w1686) -> (x*y=w1679:dbl)
                    n552 = Less?(x=w1678, y=w1684) -> (x < y?=w1683:bool)
                    n553 = Less?(x=w1679, y=w1684) -> (x < y?=w1682:bool)
                    n554 = Divide(x=w1661, y=1000.0 ("x")) -> (x/y=w1657:dbl[])
                    n555 = And(x=w1683, y=w1682) -> (x .and. y?=w1676:bool)
                    n556 = Select(t=u16 0 ("Multiplier"), s=w1676, f=u16 1 ("Multiplier")) -> (s? t:f=w1669:u16)
                    n557 = Select(t=10.0, s=w1676, f=1.0) -> (s? t:f=w1677:dbl)
                    n558 = Multiply(x=w1679, y=w1677) -> (x*y=w1671:dbl)
                    n559 = Multiply(x=w1678, y=w1677) -> (x*y=w1670:dbl)
                  }
                  frame "Mass" {
                  }
                }
              }
            }
            n560 = Index Array(array=w1561) -> (element #1=w1562:dbl, element #2=w1556:dbl)  [unwired: 2 in]
            n561 = Index Array(array=w1560) -> (element #1=w1558:dbl, element #2=w1557:dbl)  [unwired: 2 in]
            n562 = Index Array(array=w1539) -> (element #1=w1553:dbl, element #2=w1552:dbl)  [unwired: 2 in]
            n563 = Index Array(array=w1559) -> (element #1=w1555:dbl, element #2=w1554:dbl)  [unwired: 2 in]
            n564 = Bundle By Name(cluster=w1575, "Low speed (km/s)"=w1562, "High speed (km/s)"=w1556, "Window (Delta-T)"=w1565, "Lower Cutoff"=w1564, "Multiplier"=w1563, "Low Charge (fC)"=w1558, "High Charge (fC)"=w1557, "Low Mass (kg)"=w1555, "High Mass (kg)"=w1554, "Low Radius (µm)"=w1553, "High Radius (µm)"=w1552, "Exp. Voltage (MV)"=w1534) -> (w1576:T1)
            n565 = local write "PSU Calc"(w1576) -> ()
          }
          event "Accept All Particles": Value Change {
            w1703 = 10.0 ("x")
            w1709 = 0.01 ("x")
            w1710 = 200.0 ("x")
            w1715 = 0.1 ("Low speed (km/s)")
            n566 = event-data() -> ()  [unwired: 1 in, 6 out]
            n567 = property on="PSU Calc" class="Clust (strict)"(error in=w1719) -> (error out=w1718:errorcluster, "Value"=w1717:T1)  [unwired: 1 in, 1 out]
            n568 = Unbundle By Name(w1717) -> ("Low speed (km/s)"=w1714:dbl, "High speed (km/s)"=w1711:dbl, "Low Radius (µm)"=w1707:dbl, "High Radius (µm)"=w1701:dbl)
            n569 = Less?(x=w1715, y=w1714) -> (x < y?=w1716:bool)
            n570 = Select(t=w1715, s=w1716, f=w1714) -> (s? t:f=w1712:dbl)
            n571 = property on="Low speed (km/s)" class="DigNum (strict)"(error in=w1718, "Value"=w1712) -> (error out=w1706:errorcluster)  [unwired: 1 in, 1 out]
            n572 = Greater?(x=w1710, y=w1711) -> (0:w1713:bool)
            n573 = Select(t=w1710, s=w1713, f=w1711) -> (s? t:f=w1700:dbl)
            n574 = property on="High speed (km/s)" class="DigNum (strict)"(error in=w1706, "Val(Sgnl)"=w1700) -> (error out=w1705:errorcluster)  [unwired: 1 in, 1 out]
            n575 = Less?(x=w1709, y=w1707) -> (x < y?=w1708:bool)
            n576 = Select(t=w1709, s=w1708, f=w1707) -> (s? t:f=w1699:dbl)
            n577 = property on="Low Radius (µm)" class="DigNum (strict)"(error in=w1705, "Value"=w1699) -> (error out=w1704:errorcluster)  [unwired: 1 in, 1 out]
            n578 = Greater?(x=w1703, y=w1701) -> (0:w1702:bool)
            n579 = Select(t=w1703, s=w1702, f=w1701) -> (s? t:f=w1698:dbl)
            n580 = property on="High Radius (µm)" class="DigNum (strict)"(error in=w1704, "Val(Sgnl)"=w1698) -> (error out=w1697:errorcluster)  [unwired: 1 in, 1 out]
          }
        }
        n581 = Or(x="PSU update", y="OK1") -> (x .or. y?=w536:bool)
        n582 = Or(x="Cancel", y=w536) -> (x .or. y?=w532:bool)
        n583 = Not(x=w534) -> (.not. x?=w533:bool)
        n584 = Compound Arithmetic op=OR(w533, w531, w532) -> (w530:bool)
        n585 = flat-sequence {
          tunnel: [w540] -> w526
          tunnel: w525 -> [w540]
          tunnel: [w539] -> w524
          frame #0 {
            n586 = local read "PSU Calc"() -> (w539:T1)
          }
        }
        n587 = Wait Until Next ms Multiple(millisecond multiple=u32 50) -> ()  [unwired: 1 out]
      }
      "OK" <- w75
      "Cancel 2" <- w68
      n588 = case shown="False" w68 {
        tunnel: w67 -> [w114 w116]
        tunnel: [w104 w116] -> w29
        tunnel: w66 -> [w115 _]
        frame False {
          n589 = Get Date/Time In Seconds() -> (seconds since 1Jan1904=w112:timestamp)
          n590 = global write "PSU updated.vi" "PSU updated"(TRUE ("PSU updated")) -> ()
          n591 = Unbundle By Name(w115) -> ("High speed (km/s)"=w102:dbl, "Low speed (km/s)"=w101:dbl, "High Charge (fC)"=w100:dbl, "Low Charge (fC)"=w99:dbl, "High Mass (kg)"=w110:dbl, "Low Mass (kg)"=w109:dbl)
          n592 = local read "Variable 1"() -> (w108:enum32{"Velocity", "Charge", "Mass"})
          n593 = local read "Variable 2"() -> (w107:enum32{"Velocity", "Charge", "Mass"})
          n594 = call "LV_to_int_time.vi"("error in (no error)"=w114, "Time Stamp"=w112) -> ("error out"=w105:errorcluster, "Integer Time"=w113:i64)  [unwired: 7 in]
          n595 = Bundle By Name(cluster=T5 {"Integer Timestamp"=0, "Max Velocity"=0.0, "Min Velocity"=0.0, "Max Charge"=0.0, "Min Charge"=0.0, "Max Mass"=0.0, "Min Mass"=0.0, "Variable 1"=enum."Mass", "Variable 2"=enum."Mass"} ("PSU settings"), "Integer Timestamp"=w113, "Max Velocity"=w102, "Min Velocity"=w101, "Max Charge"=w100, "Min Charge"=w99, "Max Mass"=w110, "Min Mass"=w109, "Variable 1"=w108, "Variable 2"=w107) -> (w103:T5)
          n596 = call-poly "post_to_db.vi"("error in (no error)"=w105, "PSU settings"=w103) -> ("error out"=w104:errorcluster)  [unwired: 9 in]
        }
        frame True {
        }
      }
      n597 = property class="VI"(error in=w29) -> (error out=w28:errorcluster, "FP.State"=w33:T3)  [unwired: 1 in, 1 out]
      n598 = Not Equal?(x=w33, y=T3."Closed") -> (x != y?=w31:bool)
      n599 = And(x="sub vi?", y=w31) -> (x .and. y?=w34:bool)
      n600 = case shown="True" w34 {
        tunnel: w28 -> [w87 w90]
        tunnel: [w87 w89] -> w36
        tunnel: [FALSE ("sub vi?") FALSE ("sub vi?")] -> w30
        frame False {
        }
        frame True {
          n601 = invoke class="VI" method="FP.Close"(error in=w90) -> (error out=w89:errorcluster)  [unwired: 2 in, 2 out]
        }
      }
      n602 = local write "sub vi?"(w30) -> ()
    }
    frame Error {
    }
  }
  "error out" <- w10
